vi "imp_test_v10.vi"() -> ()   [LabVIEW 2014]
uses:
  <vilib>/LabVIEW Targets/FPGA/cRIO/shared/nicrio_ModuleControls/nicrio_cRIO-9237_DataRatesRing.ctl
  <vilib>/LabVIEW Targets/FPGA/cRIO/shared/nicrio_ModuleControls/nicrio_cRIO-9237_ExcitationVoltageRing.ctl
  <vilib>/rvi/FXPMathLib/FxpSinAndCos/subVIs/nifxpmath_SinAndCos_SimConfig.ctl
  <vilib>/rvi/Emulation/niFpgaGetClockAttributes.vi
  <vilib>/rvi/Emulation/niFpgaSctlEmulationGetInTimedLoop.vi
  <vilib>/rvi/Emulation/niFpgaEmulationReportErrorSimple.vi
  <vilib>/rvi/Emulation/niFpgaProcessEmulError.vi
  <vilib>/rvi/interface/RandomDataEmulation/nirviRandomDataMultiElementFPGAFIFO.vi
  <instcachedir>/0/nirviRandomDataMultiElementFPGAFIFO_AD0CFC12EF974623A9C2E4184BC062B2.lvgen/nirviRandomDataMultiElementFPGAFIFO_AD0CFC12EF974623A9C2E4184BC062B2_010.vi
  <vilib>/rvi/interface/RandomDataEmulation/niFpgaRandomDataHandleErrors.vi
  <vilib>/rvi/Emulation/niFpgaCriticalErrorInLSC.vi
  <vilib>/rvi/FXPMathLib/FxpSinAndCos/simVIs/DllFxpSinAndCosTemp_sub.vi
  <vilib>/rvi/eio/common/nirviEmuTemplateMethod_errors.vi
  <vilib>/rvi/eio/common/nirviEmuTemplatePropertySet_errors.vi
  <vilib>/rvi/DataTransferAndStorage/Container/XNode/niFpgaContainer.xnode
  <vilib>/rvi/interface/RandomDataEmulation/nirviRandomDataFpgaMultiElementTemplate.vi
  <vilib>/rvi/FXPMathLib/FxpSinAndCos/XNode/nifxpmath_SinAndCos.xnode
  <vilib>/eio/EIONode/EIONode.xnode
  <vilib>/rvi/Analysis/measure/butterworth/XNode/niFpgaButterworthFilter.xnode
  <vilib>/eio/EIOPropertyNode/EIOPropertyNode.xnode
  <vilib>/rvi/eio/common/nirviEmuTemplatePropertyGet_errors.vi
  <vilib>/rvi/eio/common/nirviEmuTemplatePropertyGet_noerrors.vi
  <vilib>/rvi/eio/common/nirviEmuTemplatePropertySet_noerrors.vi
panel:
  in  "F_Threshold_p":fxp<+,12,4>
  in  "F_Threshold_y":fxp<+,12,4>
  out "omega_y (Mavg)":fxp<+/-,36,13>
  out "Dy_d (Mavg)":fxp<+/-,36,13>
  out "omega_p (Mavg)":fxp<+/-,36,13>
  out "Dp_d (Mavg)":fxp<+/-,36,13>
  out "omega_p2 (Mavg)":fxp<+/-,36,14>
  out "Dp2_d (Mavg)":fxp<+/-,36,14>
  out "omega_y2 (Mavg)":fxp<+/-,64,27>
  out "Dy2_d (Mavg)":fxp<+/-,36,14>
  in  "mt0_y2":u32
  in  "mt0_p2":u32
  out "Dy_d (Mavg w. f.)":fxp<+/-,36,14>
  out "Dp_d (Mavg w. f.)":fxp<+/-,36,14>
  in  "Dp_d (Mavg) coeff.":i32[](array[numeric])=[946630756, 63555534]
  in  "Dy_d (Mavg) coeff.":i32[](array[numeric])=[946630756, 63555534]
  out "omega_y (Mavg w. f.)":fxp<+/-,36,14>
  in  "omega_y(Mavg) coeff.":i32[](array[numeric])=[946630756, 63555534]
  out "omega_p (Mavg w. f)":fxp<+/-,36,14>
  in  "omega_P(Mavg) coeff.":i32[](array[numeric])=[946630756, 63555534]
  in  "FIFO":i16(ring) items=["Pitch_F+P", "imp ctrl", "Yaw_F+P"]
  out "PID (kHz)":fxp<+/-,20,10>
  in  "Set 6":bool
  in  "Set 5":bool
  in  "Set 4":bool
  in  "Set 3":bool
  in  "Set 2":bool
  in  "Set 1":bool
  out "Dy1_d (T)":fxp<+/-,36,13>
  out "omega_y1 (T)":fxp<+/-,36,13>
  out "Dp1_d (T)":fxp<+/-,36,13>
  out "omega_p1 (T)":fxp<+/-,36,13>
  out "Dy2_d (T)":fxp<+/-,36,13>
  out "Dp2_d (T)":fxp<+/-,36,13>
  out "omega_y2 (T)":fxp<+/-,36,13>
  out "omega_p2 (T)":fxp<+/-,36,13>
  out "mt_omega_y2":u32
  out "mt_omega_p2":u32
  out "rad_y2":fxp<+/-,33,20>
  out "D_y2":fxp<+/-,32,7>
  out "rad_y1":fxp<+/-,33,20>
  out "D_y1":fxp<+/-,32,7>
  out "Encoder Position_y1":i32
  out "Encoder Position_y2":i32
  out "Encoder Position_p2":i32
  out "D_p2":fxp<+/-,32,7>
  out "rad_p2":fxp<+/-,33,20>
  out "D_p1":fxp<+/-,32,7>
  out "rad_p1":fxp<+/-,33,20>
  out "Encoder Position_p1":i32
  in  "Mag. factor_y":fxp<+/-,20,3>
  in  "Mag. encoder_y":bool
  out "omega_y (rad/s)":fxp<+/-,36,13>
  out "Dy_d (mm/s)":fxp<+/-,36,13>
  in  "Vy. Est.":i16(ring) items=["T", "Mavg", "Mavg w. f."]
  out "omega_y1 (Mavg)":fxp<+/-,36,14>
  out "Dy1_d (Mavg)":fxp<+/-,36,14>
  in  "Dy_d_M_avg_Tc (uSec)":i32
  out "Dp1_d (Mavg)":fxp<+/-,36,14>
  out "omega_p1 (Mavg)":fxp<+/-,36,14>
  in  "Dp_d_M_avg_Tc (uSec)":i32
  out "Dp_d (T)":fxp<+/-,36,13>
  out "omega_p (T)":fxp<+/-,36,13>
  in  "Vp. Est.":i16(ring) items=["T", "Mavg", "Mavg w. f."]
  in  "Mag. factor_p":fxp<+/-,20,3>
  in  "Mag. encoder_p":bool
  in  "Belt_out_p":fxp<+/-,7,7>
  in  "Belt_in_p":fxp<+/-,6,6>
  in  "Belt_out_y":fxp<+/-,7,7>
  in  "Belt_in_y":fxp<+/-,6,6>
  out "Fp_dc":fxp<+/-,32,10>
  out "Fy_dc":fxp<+/-,32,10>
  in  "Zero_y":bool
  in  "Zero_p":bool
  in  "mt0_p1":u32
  in  "Encoder reset":bool
  out "fpt_d":fxp<+/-,36,18>
  out "Dp_error_dd":fxp<+/-,36,16>
  out "Dp_error_d":fxp<+/-,33,8>
  in  "Dp_dd coeff.":i32[](array[numeric])=[946630756, 63555534]
  out "Dp_dd":fxp<+/-,36,25>
  out "dFp_PID":fxp<+/-,36,18>
  in  "dFp_PID coeff.":i32[](array[numeric])=[946630756, 63555534]
  out "fpt_i":fxp<+/-,34,18>
  in  "Bv_p":fxp<+/-,22,8>
  in  "Kv_p":fxp<+/-,22,8>
  out "Dp_error":fxp<+/-,22,7>
  out "Dpr_sin":fxp<+/-,22,7>
  in  "Sin offset_p":fxp<+/-,22,7>
  in  "Sin magnitude_p":fxp<+/-,21,6>
  out "Dpr_sin_dd":fxp<+/-,35,20>
  out "Dpr_sin_d":fxp<+/-,33,15>
  out "Sin omega_p":fxp<+/-,34,9>
  in  "Sin wave freq._p (Hz)":fxp<+/-,32,6>
  in  "Dpr_step":fxp<+/-,22,7>
  out "Dpr_for":fxp<+/-,22,7>
  in  "Command_p":i16(ring) items=["Step", "Sine"]
  in  "Ki_p":fxp<+/-,30,9>
  out "Fp_PID":fxp<+/-,36,16>
  in  "fp_tolorance":fxp<+,22,6>
  out "fp_tilde":fxp<+/-,33,10>
  in  "Kd_p":fxp<+/-,30,9>
  in  "Kp_p":fxp<+/-,32,13>
  out "Fr_p":fxp<+/-,32,10>
  in  "S/F coeff_p":fxp<+/-,25,-10>
  in  "S/F coeff_y":fxp<+/-,25,-10>
  out "va_p":fxp<+/-,36,7>
  out "vb_p":fxp<+/-,37,8>
  out "vq_p_F":fxp<+/-,20,5> format="%.57g"
  out "vd_p_F":fxp<+/-,20,5>
  in  "dFp_add":bool
  in  "Stop motor_p":bool
  out "Force_p":fxp<+/-,32,10>
  in  "Strain selection_p":i16(ring) items=["Raw", "Avg.8", "Avg.8 w. filter"]
  out "Strain_p (Avg8 w. f)":fxp<+/-,36,8>
  in  "Strain_p Avg.8 coeff.":i32[](array[numeric])=[946630756, 63555534]
  out "Strain_p (Avg8)":fxp<+/-,36,4>
  out "Raw Strain_p":fxp<+/-,36,4>
  out "Mod6/AI3":fxp<+/-,36,4>
  in  "Strain gage reset_p":bool
  out "Dp_d (mm/s)":fxp<+/-,36,13>
  out "omega_p (rad/s)":fxp<+/-,36,13>
  out "mt_omega_p1":u32
  out "rad_p(NrTheta)":fxp<+/-,33,20>
  out "D_p(mm)":fxp<+/-,32,7>
  out "Encoder Position_p":i32
  in  "Encoder reset_p":bool
  out "Strain_y (Avg8 w. f)":fxp<+/-,36,8>
  in  "Strain_y Avg8 coeff.":i32[](array[numeric])=[-898916953, 1957103773, 3888751]
  out "Dyr_for":fxp<+/-,22,7>
  in  "Command_y":i16(ring) items=["Step", "Sine"]
  out "Strain_y (Avg8)":fxp<+/-,36,4>
  in  "Strain selection_y":i16(ring) items=["Raw", "Avg.8", "Avg.8 w. filter"]
  out "vb_y":fxp<+/-,38,8>
  out "va_y":fxp<+/-,38,8>
  out "fyt_d":fxp<+/-,36,18>
  out "Fr_y":fxp<+/-,32,10>
  in  "Bv_y":fxp<+/-,22,8>
  out "Dy_error_dd":fxp<+/-,36,16>
  out "Dy_error_d":fxp<+/-,33,8>
  in  "Kv_y":fxp<+/-,22,8>
  out "Dy_error":fxp<+/-,22,7>
  out "Dyr_sin_dd":fxp<+/-,35,20>
  out "Dyr_sin_d":fxp<+/-,33,15>
  out "Sin omega_y":fxp<+/-,34,9>
  out "Dyr_sin":fxp<+/-,22,7>
  in  "Sin offset_y":fxp<+/-,22,7>
  in  "Sin magnitude_y":fxp<+/-,21,6>
  out "Time now(s)":fxp<+,52,14>
  in  "Sin wave freq._y (Hz)":fxp<+/-,32,6>
  in  "Dyr_step":fxp<+/-,22,7>
  in  "Drive mode":i16(ring) items=["Backward", "Forward"]
  out "Dy_dd":fxp<+/-,36,25>
  in  "Dy_dd coeff.":i32[](array[numeric])=[946630756, 63555534]
  out "dFy_PID":fxp<+/-,36,18>
  in  "dFy_PID coeff.":i32[](array[numeric])=[946630756, 63555534]
  out "fyt_i":fxp<+/-,36,16>
  out "Fy_PID":fxp<+/-,36,16>
  in  "fy_tolorance":fxp<+,22,6>
  in  "Ki_y":fxp<+/-,30,9>
  in  "Kd_y":fxp<+/-,30,9>
  out "fy_tilde":fxp<+/-,32,10>
  in  "Kp_y":fxp<+/-,32,13>
  out "vq_y_F":fxp<+/-,20,5> format="%.57g"
  out "vd_y_F":fxp<+/-,20,5>
  in  "dFy_add":bool
  in  "Stop motor_y":bool
  out "Dy_d (T)":fxp<+/-,36,13>
  out "omega_y (T)":fxp<+/-,36,13>
  in  "mt0_y1":u32
  out "mt_omega_y1":u32
  out "rad_y(NrTheta)":fxp<+/-,33,20>
  out "D_y(mm)":fxp<+/-,32,7>
  out "Encoder Position_y":i32
  in  "Encoder reset_y":bool
  in  "Ini coe.":bool
  out "Loop rate (kHz)":fxp<+/-,36,7>
  out "Force_y":fxp<+/-,32,10>
  out "Raw Strain_y":fxp<+/-,36,4>
  in  "Strain gage reset_y":bool
  in  "Stop (Strain)":bool
  out "Mod6/AI2":fxp<+/-,36,4>
  in  "Excitation Voltage":T1 items=["2.5 Volts", "3.3 Volts", "5.0 Volts", "10.0 Volts", "External Excitation"]
  in  "Data Rate":T2=1 items=["50.000 kS/s (NI 9237)"=1, "25.000 kS/s (NI 9237)"=2, "16.667 kS/s (NI 9237)"=3, "12.500 kS/s (NI 9237)"=4, "10.000 kS/s (NI 9237)"=5, "8.333 kS/s (NI 9237)"=6, "7.143 kS/s (NI 9237)"=7, "6.250 kS/s (NI 9237)"=8, "5.556 kS/s (NI 9237)"=9, "5.000 kS/s (NI 9237)"=10, "4.545 kS/s (NI 9237)"=11, "4.167 kS/s (NI 9237)"=12, "3.846 kS/s (NI 9237)"=13, "3.571 kS/s (NI 9237)"=14, "3.333 kS/s (NI 9237)"=15, "3.125 kS/s (NI 9237)"=16, "2.941 kS/s (NI 9237)"=17, "2.778 kS/s (NI 9237)"=18, "2.632 kS/s (NI 9237)"=19, "2.500 kS/s (NI 9237)"=20, "2.381 kS/s (NI 9237)"=21, "2.273 kS/s (NI 9237)"=22, "2.174 kS/s (NI 9237)"=23, "2.083 kS/s (NI 9237)"=24, "2.000 kS/s (NI 9237)"=25, "1.923 kS/s (NI 9237)"=26, "1.852 kS/s (NI 9237)"=27, "1.786 kS/s (NI 9237)"=28, "1.724 kS/s (NI 9237)"=29, "1.667 kS/s (NI 9237)"=30, "1.613 kS/s (NI 9237)"=31]
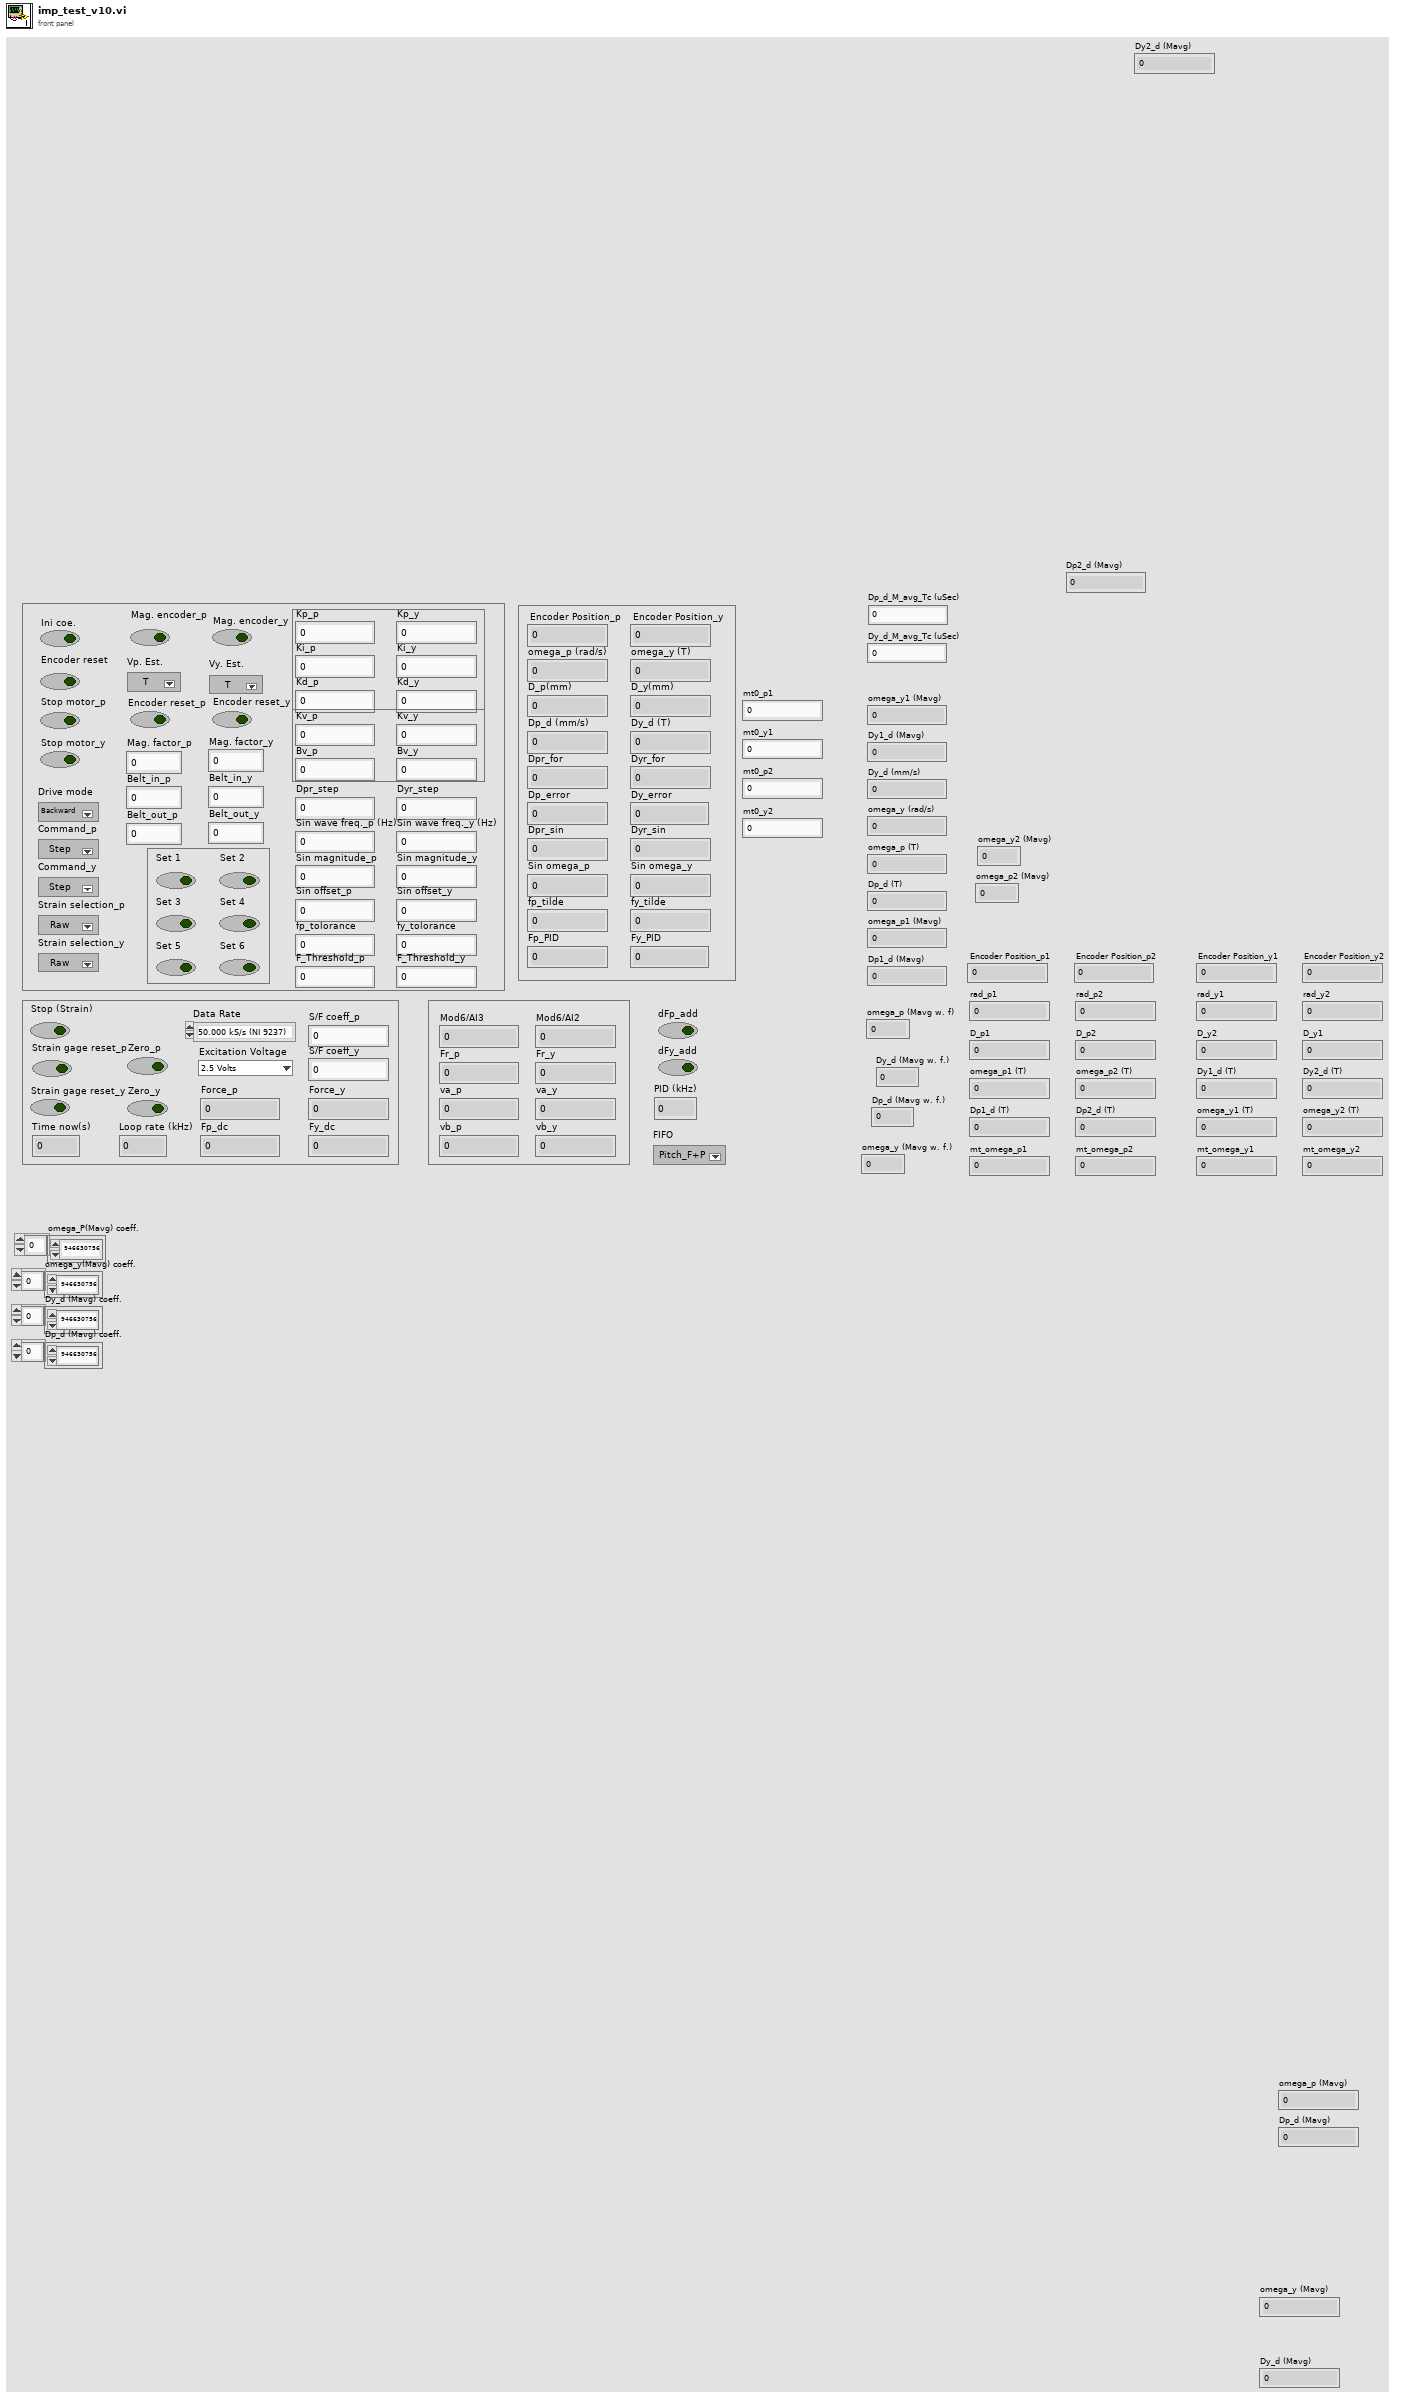
[diagram p1: front panel]
types:
  T1 = typedef "nicrio_cRIO-9237_ExcitationVoltageRing.ctl" = u8
  T2 = typedef "nicrio_cRIO-9237_DataRatesRing.ctl" = u8
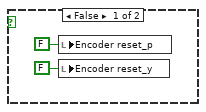
[diagram p12: hidden frame]
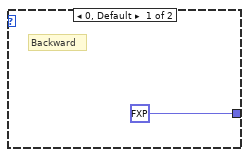
[diagram p13: hidden frame]
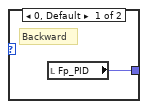
[diagram p14: hidden frame]
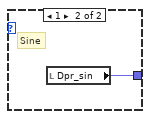
[diagram p15: hidden frame]
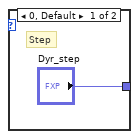
[diagram p16: hidden frame]
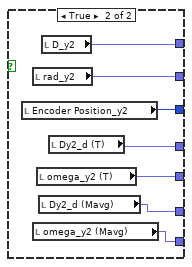
[diagram p17: hidden frame]
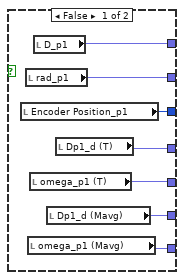
[diagram p18: hidden frame]
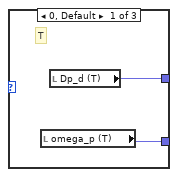
[diagram p19: hidden frame]
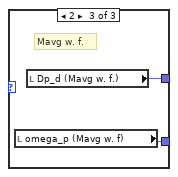
[diagram p20: hidden frame]
diagram:
  w2 = 25
  w5 = i16 25
  w13 = 25
  w16 = 25
  w21 = TRUE ("Half-Bridge Enable")
  # "rad_x2那邊:數據叫出來/8才會和馬達編碼器的rad一樣??"
  # "Encoder 4096ppr\nomega = 61359.2315154/mt\nomega0 = 2*pi/4096 (rad/s)"
  # "Encoder 800ppr\nomega = 314159.265359/mt\nomega0 = 2*pi/800 (rad/s)"
  # "v9\nKp改32/13\nKd改30/9\nKo改30/9"
  # "Resolutuin of Mag. Encoder = 4096*(F_mag)"
  # "use Mavg method to estimate omega or velocity from magnetic encoder"
  # "為什麼要寫兩個迴圈?\nv9後已修正"
  # "Dr_dd ?"
  # "Dr_d ?"
  n1 = xnode "FPGA I/O Property Node"("error in"=errorcluster {"status"=FALSE, "code"=0, "source"=""}, "Data Rate"="Data Rate", "Excitation Voltage"="Excitation Voltage") -> ("error out"=w26:errorcluster)  [unwired: 1 in, 1 out]
  n2 = xnode "FPGA I/O Property Node"("error in"=w26, "Half-Bridge Enable"=w21) -> ("error out"=w19:errorcluster)  [unwired: 1 in, 1 out]
  n3 = xnode "FPGA I/O Property Node"("Half-Bridge Enable"=w21) -> ("error out"=w18:errorcluster)  [unwired: 2 in, 1 out]
  n4 = Merge Errors(w19, w18) -> (w20:errorcluster)
  n5 = xnode "FPGA I/O Node"("error in"=w20, "Mod6/Start"=TRUE) -> ("error out"=w24:errorcluster)  [unwired: 1 in, 1 out]
  n6 = while "AO_p" {
    stop <- FALSE stop-if-true
    n7 = flat-sequence {
      frame #0 {
        n8 = local read "rad_p(NrTheta)"() -> (w41:fxp<+/-,33,20>)
        n9 = local read "vq_p_F"() -> (w42:fxp<+/-,20,5>)
        n10 = local read "vd_p_F"() -> (w44:fxp<+/-,20,5>)
        n11 = Select(t=fxp<+/-,20,5> 0.0, s="Stop motor_p", f=w44) -> (s? t:f=w33:fxp<+/-,20,5>)
        n12 = Select(t=fxp<+,1,1> 0.0, s="Stop motor_p", f=w42) -> (s? t:f=w32:fxp<+/-,20,5>)
        n13 = xnode "High Throughput Sine & Cosine"("x (pi)"=w41) -> ("sin(x)"=w35:fxp<+/-,16,2>, "cos(x)"=w34:fxp<+/-,16,2>)
        n14 = Negate(x=w32) -> (-x=w40:fxp<+/-,21,6>)
        n15 = Multiply(x=w33, y=w35) -> (x*y=w39:fxp<+/-,36,7>)
        n16 = Multiply(x=w33, y=w34) -> (x*y=w37:fxp<+/-,36,7>)
        n17 = Multiply(x=w34, y=w32) -> (x*y=w38:fxp<+/-,36,7>)
        n18 = Multiply(x=w35, y=w40) -> (x*y=w36:fxp<+/-,35,6>)
        n19 = Add(x=w39, y=w38) -> (x+y=→"vb_p":fxp<+/-,37,8>)
        n20 = Add(x=w37, y=w36) -> (x+y=→"va_p":fxp<+/-,36,7>)
      }
      frame #1 {
        n21 = local read "Encoder reset_p"() -> (w77:bool)
        n22 = local read "vb_p"() -> (w78:fxp<+/-,37,8>)
        n23 = local read "va_p"() -> (w79:fxp<+/-,36,7>)
        n24 = Select(t=fxp<+,2,2> 3.0, s=w77, f=w79) -> (s? t:f=w85:fxp<+/-,36,7>)
        n25 = Select(t=fxp<+,1,1> 0.0, s=w77, f=w78) -> (s? t:f=w84:fxp<+/-,37,8>)
        n26 = Multiply(x=w85, y=fxp<+/-,1,0> -0.5) -> (x*y=w80:fxp<+/-,36,6>)
        n27 = Multiply(x=w84, y=fxp<+/-,1,0> -0.5) -> (x*y=w81:fxp<+/-,36,6>)
        n28 = xnode "FPGA I/O Node"("Mod8/AO0"=w80, "Mod8/AO1"=w81) -> ()  [unwired: 2 in, 2 out]
      }
    }
  }
  n29 = while "AO_y" {
    stop <- FALSE stop-if-true
    n30 = flat-sequence {
      frame #0 {
        n31 = local read "rad_y(NrTheta)"() -> (w105:fxp<+/-,33,20>)
        n32 = local read "vd_y_F"() -> (w103:fxp<+/-,20,5>)
        n33 = local read "vq_y_F"() -> (w102:fxp<+/-,20,5>)
        n34 = Select(t=fxp<+/-,20,5> 0.0, s="Stop motor_y", f=w103) -> (s? t:f=w97:fxp<+/-,20,5>)
        n35 = Select(t=fxp<+/-,20,5> 0.0, s="Stop motor_y", f=w102) -> (s? t:f=w96:fxp<+/-,20,5>)
        n36 = xnode "High Throughput Sine & Cosine"("x (pi)"=w105) -> ("sin(x)"=w99:fxp<+/-,17,2>, "cos(x)"=w98:fxp<+/-,17,2>)
        n37 = Negate(x=w96) -> (-x=w95:fxp<+/-,21,6>)
        n38 = Multiply(x=w97, y=w99) -> (x*y=w94:fxp<+/-,37,7>)
        n39 = Multiply(x=w97, y=w98) -> (x*y=w92:fxp<+/-,37,7>)
        n40 = Multiply(x=w98, y=w96) -> (x*y=w93:fxp<+/-,37,7>)
        n41 = Multiply(x=w99, y=w95) -> (x*y=w91:fxp<+/-,36,6>)
        n42 = Add(x=w94, y=w93) -> (x+y=→"vb_y":fxp<+/-,38,8>)
        n43 = Add(x=w92, y=w91) -> (x+y=→"va_y":fxp<+/-,37,7>)
      }
      frame #1 {
        n44 = local read "Encoder reset_y"() -> (w138:bool)
        n45 = local read "va_y"() -> (w137:fxp<+/-,38,8>)
        n46 = local read "vb_y"() -> (w136:fxp<+/-,38,8>)
        n47 = Select(t=fxp<+,2,2> 3.0, s=w138, f=w137) -> (s? t:f=w142:fxp<+/-,38,8>)
        n48 = Select(t=fxp<+,1,1> 0.0, s=w138, f=w136) -> (s? t:f=w141:fxp<+/-,38,8>)
        n49 = Multiply(x=w142, y=fxp<+/-,1,0> -0.5) -> (x*y=w145:fxp<+/-,39,8>)
        n50 = Multiply(x=w141, y=fxp<+/-,1,0> -0.5) -> (x*y=w146:fxp<+/-,37,6>)
        n51 = xnode "FPGA I/O Node"("Mod8/AO2"=w145, "Mod8/AO3"=w146) -> ()  [unwired: 2 in, 2 out]
      }
    }
  }
  n52 = while "Selection" {
    stop <- FALSE stop-if-true
    # "T = Mag. encoder\nF = Motor encoder"
    n53 = case shown="2" "Strain selection_y" {
      tunnel: [w229 w230 w231] -> w182
      frame 0, Default {
        n54 = local read "Raw Strain_y"() -> (w229:fxp<+/-,36,4>)
      }
      frame 1 {
        n55 = local read "Strain_y (Avg8)"() -> (w230:fxp<+/-,36,4>)
      }
      frame 2 {
        n56 = local read "Strain_y (Avg8 w. f)"() -> (w231:fxp<+/-,36,8>)
      }
    }
    n57 = case shown="1" "Vp. Est." {
      tunnel: [w213 w214 w217] -> w165
      tunnel: [w212 w215 w216] -> w166
      frame 0, Default {
        # "T"
        n58 = local read "omega_p (T)"() -> (w213:fxp<+/-,36,13>)
        n59 = local read "Dp_d (T)"() -> (w212:fxp<+/-,36,13>)
      }
      frame 1 {
        # "Mavg"
        n60 = local read "omega_p (Mavg)"() -> (w214:fxp<+/-,36,13>)
        n61 = local read "Dp_d (Mavg)"() -> (w215:fxp<+/-,36,13>)
      }
      frame 2 {
        # "Mavg w. f."
        n62 = local read "omega_p (Mavg w. f)"() -> (w217:fxp<+/-,36,14>)
        n63 = local read "Dp_d (Mavg w. f.)"() -> (w216:fxp<+/-,36,14>)
      }
    }
    "Dp_d (mm/s)" <- w166
    "omega_p (rad/s)" <- w165
    n64 = Divide(x=w182, y="S/F coeff_y") -> (x/y=w175:fxp<+/-,32,10>)
    n65 = case shown="True" "Zero_y" {
      tunnel: w175 -> [_ w225]
      frame False {
      }
      frame True {
        "Fy_dc" <- w225
      }
    }
    n66 = local read "Fy_dc"() -> (w176:fxp<+/-,32,10>)
    n67 = Subtract(x=w175, y=w176) -> (x-y=→"Force_y":fxp<+/-,33,11>)
    n68 = case shown="2" "Strain selection_p" {
      tunnel: [w226 w227 w228] -> w180
      frame 0, Default {
        n69 = local read "Raw Strain_p"() -> (w226:fxp<+/-,36,4>)
      }
      frame 1 {
        n70 = local read "Strain_p (Avg8)"() -> (w227:fxp<+/-,36,4>)
      }
      frame 2 {
        n71 = local read "Strain_p (Avg8 w. f)"() -> (w228:fxp<+/-,36,8>)
      }
    }
    n72 = case shown="1" "Vy. Est." {
      tunnel: [w219 w221 w223] -> w168
      tunnel: [w218 w220 w222] -> w169
      frame 0, Default {
        # "T"
        n73 = local read "omega_y (T)"() -> (w218:fxp<+/-,36,13>)
        n74 = local read "Dy_d (T)"() -> (w219:fxp<+/-,36,13>)
      }
      frame 1 {
        # "Mavg"
        n75 = local read "omega_y (Mavg)"() -> (w220:fxp<+/-,36,13>)
        n76 = local read "Dy_d (Mavg)"() -> (w221:fxp<+/-,36,13>)
      }
      frame 2 {
        # "Mavg w. f."
        n77 = local read "omega_y (Mavg w. f.)"() -> (w222:fxp<+/-,36,14>)
        n78 = local read "Dy_d (Mavg w. f.)"() -> (w223:fxp<+/-,36,14>)
      }
    }
    "Dy_d (mm/s)" <- w168
    "omega_y (rad/s)" <- w169
    n79 = Divide(x=w180, y="S/F coeff_p") -> (x/y=w172:fxp<+/-,32,10>)
    n80 = case shown="True" "Zero_p" {
      tunnel: w172 -> [_ w224]
      frame False {
      }
      frame True {
        "Fp_dc" <- w224
      }
    }
    n81 = local read "Fp_dc"() -> (w170:fxp<+/-,32,10>)
    n82 = Subtract(x=w172, y=w170) -> (x-y=→"Force_p":fxp<+/-,33,11>)
    n83 = case shown="False" "Mag. encoder_y" {
      tunnel: [w190 w196] -> w156
      tunnel: [w189 w197] -> w157
      tunnel: [w188 w195] -> w159
      tunnel: [w186 w194] -> w153
      tunnel: [w187 w193] -> w152
      tunnel: [w185 w192] -> w148
      tunnel: [w184 w191] -> w147
      frame False {
        n84 = local read "Encoder Position_y1"() -> (w188:i32)
        n85 = local read "omega_y1 (Mavg)"() -> (w184:fxp<+/-,36,14>)
        n86 = local read "Dy1_d (Mavg)"() -> (w185:fxp<+/-,36,14>)
        n87 = local read "rad_y1"() -> (w190:fxp<+/-,33,20>)
        n88 = local read "omega_y1 (T)"() -> (w186:fxp<+/-,36,13>)
        n89 = local read "D_y1"() -> (w189:fxp<+/-,32,7>)
        n90 = local read "Dy1_d (T)"() -> (w187:fxp<+/-,36,13>)
      }
      frame True {
        n91 = local read "Encoder Position_y2"() -> (w195:i32)
        n92 = local read "rad_y2"() -> (w196:fxp<+/-,33,20>)
        n93 = local read "omega_y2 (Mavg)"() -> (w191:fxp<+/-,64,27>)
        n94 = local read "omega_y2 (T)"() -> (w194:fxp<+/-,36,13>)
        n95 = local read "Dy2_d (Mavg)"() -> (w192:fxp<+/-,36,14>)
        n96 = local read "D_y2"() -> (w197:fxp<+/-,32,7>)
        n97 = local read "Dy2_d (T)"() -> (w193:fxp<+/-,36,13>)
      }
    }
    "D_y(mm)" <- w157
    "rad_y(NrTheta)" <- w156
    "Encoder Position_y" <- w159
    "Dy_d (T)" <- w152
    "omega_y (T)" <- w153
    "Dy_d (Mavg)" <- w148
    "omega_y (Mavg)" <- w147
    n98 = case shown="True" "Mag. encoder_p" {
      tunnel: [w204 w211] -> w161
      tunnel: [w203 w210] -> w162
      tunnel: [w202 w209] -> w163
      tunnel: [w200 w208] -> w155
      tunnel: [w201 w207] -> w154
      tunnel: [w199 w205] -> w151
      tunnel: [w198 w206] -> w150
      frame False {
        n99 = local read "Encoder Position_p1"() -> (w202:i32)
        n100 = local read "rad_p1"() -> (w203:fxp<+/-,33,20>)
        n101 = local read "omega_p1 (Mavg)"() -> (w198:fxp<+/-,36,14>)
        n102 = local read "omega_p1 (T)"() -> (w200:fxp<+/-,36,13>)
        n103 = local read "D_p1"() -> (w204:fxp<+/-,32,7>)
        n104 = local read "Dp1_d (Mavg)"() -> (w199:fxp<+/-,36,14>)
        n105 = local read "Dp1_d (T)"() -> (w201:fxp<+/-,36,13>)
      }
      frame True {
        n106 = local read "Encoder Position_p2"() -> (w209:i32)
        n107 = local read "omega_p2 (Mavg)"() -> (w206:fxp<+/-,36,14>)
        n108 = local read "rad_p2"() -> (w210:fxp<+/-,33,20>)
        n109 = local read "D_p2"() -> (w211:fxp<+/-,32,7>)
        n110 = local read "Dp2_d (Mavg)"() -> (w205:fxp<+/-,36,14>)
        n111 = local read "omega_p2 (T)"() -> (w208:fxp<+/-,36,13>)
        n112 = local read "Dp2_d (T)"() -> (w207:fxp<+/-,36,13>)
      }
    }
    "D_p(mm)" <- w161
    "rad_p(NrTheta)" <- w162
    "Encoder Position_p" <- w163
    "Dp_d (T)" <- w154
    "omega_p (T)" <- w155
    "Dp_d (Mavg)" <- w151
    "omega_p (Mavg)" <- w150
  }
  n113 = while "Quadrature drive_y" {
    stop <- FALSE stop-if-true
    n114 = local read "Drive mode"() -> (w233:i16)
    n115 = case shown="1" w233 {
      tunnel: [w243 w244] -> w232
      frame 0, Default {
        # "Backward"
        n116 = local read "Fy_PID"() -> (w243:fxp<+/-,36,16>)
      }
      frame 1 {
        # "Forward"
        n117 = local read "Fr_y"() -> (w244:fxp<+/-,32,10>)
      }
    }
    n118 = local read "dFy_PID"() -> (w236:fxp<+/-,36,18>)
    n119 = local read "omega_y (rad/s)"() -> (w242:fxp<+/-,36,13>)
    n120 = Select(t=w236, s="dFy_add", f=fxp<+,1,1> 0.0) -> (s? t:f=w239:fxp<+/-,36,18>)
    n121 = call "Oriental_step_motor_PKP225.vi"("F_Threshold"="F_Threshold_y", "dFmr"=w239, "omega"=w242, "Fmr"=w232) -> ("vq_F"=→"vq_y_F":fxp<+/-,36,9>, "vd_F"=→"vd_y_F":fxp<+/-,36,9>)  [unwired: 6 in]
  }
  n122 = while "Encoder_p" {
    shift-right: [w282] -> _
    shift-left: _ -> [w281]
    shift-right: [w283] -> _
    shift-left: _ -> [w280]
    shift-right: [w277] -> _
    shift-left: _ -> [w279]
    shift-right: [w268] -> _
    shift-left: _ -> [w267]
    shift-right: [w269] -> _
    shift-left: _ -> [w270]
    shift-right: [w264] -> _
    shift-left: _ -> [w265]
    stop <- FALSE stop-if-true
    w260 = fxp<+/-,20,-5> 0.00048828125  # L/4096
    w258 = fxp<+/-,16,1> 0.0244140625  # 2*50/4096)
    w276 = fxp<+/-,20,-5> 0.002499997615814209  # L/800
    w250 = fxp<+/-,16,1> 0.125  # 2*50/800
    n123 = xnode "FPGA I/O Node"() -> ("Mod7/DIO0"=w285:bool, "Mod7/DIO1"=w284:bool)  [unwired: 2 in, 2 out]
    n124 = xnode "FPGA I/O Node"() -> ("Mod7/DIO4"=w272:bool, "Mod7/DIO5"=w271:bool)  [unwired: 2 in, 2 out]
    n125 = local read "Encoder reset_p"() -> (w266:bool)
    n126 = call "encoder_sub.vi"("A_pre"=w281, "B_pre"=w280, "Encoder Position_pre"=w279, "A input"=w285, "Encoder Position Reset"="Encoder reset_p", "B input"=w284) -> ("A"=w282:bool, "B"=w283:bool, "Encoder Position (Counts)"=w277:i32)  [unwired: 19 in]
    "Encoder Position_p1" <- w277
    n127 = call "encoder_sub.vi"("A_pre"=w267, "B_pre"=w270, "Encoder Position_pre"=w265, "A input"=w272, "Encoder Position Reset"=w266, "B input"=w271) -> ("A"=w268:bool, "B"=w269:bool, "Encoder Position (Counts)"=w264:i32)  [unwired: 19 in]
    "Encoder Position_p2" <- w264
    n128 = local read "Belt_in_p"() -> (w275:fxp<+/-,6,6>)
    n129 = local read "Belt_in_p"() -> (w261:fxp<+/-,6,6>)
    n130 = local read "Belt_out_p"() -> (w273:fxp<+/-,7,7>)
    n131 = To Fixed-Point(number=w264) -> (fixed-point=w246:fxp<+/-,32,32>)  [unwired: 1 in]
    n132 = To Fixed-Point(number=w277) -> (fixed-point=w251:fxp<+/-,32,32>)  [unwired: 1 in]
    n133 = local read "Belt_out_p"() -> (w263:fxp<+/-,7,7>)
    n134 = local read "Mag. factor_p"() -> (w257:fxp<+/-,20,3>)
    n135 = Divide(x=w260, y="Mag. factor_p") -> (x/y=w259:fxp<+/-,41,13>)
    n136 = Multiply(x=w276, y=w275) -> (x*y=w274:fxp<+/-,26,1>)
    n137 = Multiply(x=w259, y=w261) -> (x*y=w262:fxp<+/-,46,18>)
    n138 = Divide(x=w274, y=w273) -> (x/y=w253:fxp<+/-,33,1>)
    n139 = Divide(x=w262, y=w263) -> (x/y=w248:fxp<+/-,53,18>)
    n140 = Divide(x=w258, y=w257) -> (x/y=w245:fxp<+/-,37,5>)
    n141 = Multiply(x=w251, y=w250) -> (x*y=→"rad_p1":fxp<+/-,33,20>)
    n142 = Multiply(x=w248, y=w246) -> (x*y=→"D_p2":fxp<+/-,37,7>)
    n143 = Multiply(x=w246, y=w245) -> (x*y=→"rad_p2":fxp<+/-,46,16>)
    n144 = Multiply(x=w253, y=w251) -> (x*y=→"D_p1":fxp<+/-,32,7>)
  }
  n145 = while "Integral and derivative" {
    shift-right: [w341] -> _
    shift-left: _ -> [w340]
    shift-right: [w333] -> _
    shift-left: _ -> [w332]
    shift-right: [w343] -> _
    shift-left: _ -> [w344]
    shift-right: [w323] -> _
    shift-left: _ -> [w322]
    shift-right: [w309] -> _
    shift-left: _ -> [w312]
    shift-right: [w302] -> _
    shift-left: _ -> [w301]
    shift-right: [w296] -> _
    shift-left: _ -> [w295]
    shift-right: [w291] -> _
    shift-left: _ -> [w292]
    stop <- FALSE stop-if-true
    # "Pitch"
    # "Yaw"
    n146 = local read "Dp_d (mm/s)"() -> (w291:fxp<+/-,36,13>)
    n147 = local read "Dy_d (mm/s)"() -> (w323:fxp<+/-,36,13>)
    n148 = local read "Fp_PID"() -> (w296:fxp<+/-,36,16>)
    n149 = local read "fp_tilde"() -> (w313:fxp<+/-,33,10>)
    n150 = local read "fp_tolorance"() -> (w316:fxp<+,22,6>)
    n151 = local read "fy_tolorance"() -> (w319:fxp<+,22,6>)
    n152 = local read "fy_tilde"() -> (w345:fxp<+/-,32,10>)
    n153 = local read "Fy_PID"() -> (w343:fxp<+/-,36,16>)
    n154 = Subtract(x=w296, y=w295) -> (x-y=w300:fxp<+/-,37,17>)
    n155 = Subtract(x=w291, y=w292) -> (x-y=w293:fxp<+/-,37,14>)
    n156 = Absolute Value(x=w313) -> (abs(x)=w317:fxp<+,33,10>)
    n157 = Absolute Value(x=w345) -> (abs(x)=w347:fxp<+,32,10>)
    n158 = Subtract(x=w343, y=w344) -> (x-y=w331:fxp<+/-,37,17>)
    n159 = Subtract(x=w323, y=w322) -> (x-y=w325:fxp<+/-,36,11>)
    n160 = Greater?(x=w347, y=w319) -> (0:w348:bool)
    n161 = Greater?(x=w317, y=w316) -> (0:w315:bool)
    n162 = Multiply(x=fxp<+,7,10> 1000.0, y=w300) -> (x*y=w298:fxp<+/-,32,18>)
    n163 = Multiply(x=fxp<+,7,10> 1000.0, y=w293) -> (x*y=w289:fxp<+/-,36,21>)
    n164 = local read "Stop motor_y"() -> (w334:bool)
    n165 = local read "Stop motor_p"() -> (w304:bool)
    n166 = Select(t=w345, s=w348, f=fxp<+/-,33,11> 0.0) -> (s? t:f=w341:fxp<+/-,33,11>)
    n167 = Select(t=w313, s=w315, f=fxp<+,1,1> 0.0) -> (s? t:f=w309:fxp<+/-,33,10>)
    n168 = Multiply(x=fxp<+,7,10> 1000.0, y=w325) -> (x*y=w324:fxp<+/-,36,21>)
    n169 = xnode "Butterworth Filter"("input data"=w298, "scaled coefficients"="dFp_PID coeff.") -> ("output data"=→"dFp_PID":fxp<+/-,36,22>)  [unwired: 1 in]
    n170 = xnode "Butterworth Filter"("input data"=w289, "scaled coefficients"="Dp_dd coeff.") -> ("output data"=→"Dp_dd":fxp<+/-,36,25>)  [unwired: 1 in]
    n171 = Multiply(x=fxp<+,7,10> 1000.0, y=w331) -> (x*y=w328:fxp<+/-,32,18>)
    n172 = Add(x=w340, y=w341) -> (x+y=w346:fxp<+/-,34,12>)
    n173 = Multiply(x=w312, y=w309) -> (x*y=w311:fxp<+/-,34,12>)
    n174 = xnode "Butterworth Filter"("input data"=w324, "scaled coefficients"="Dy_dd coeff.") -> ("output data"=→"Dy_dd":fxp<+/-,36,25>)  [unwired: 1 in]
    n175 = Multiply(x=fxp<+/-,30,12> 0.000499725341796875, y=w346) -> (x*y=w339:fxp<+/-,34,10>)
    n176 = Multiply(x=fxp<+/-,30,12> 0.000499725341796875, y=w311) -> (x*y=w308:fxp<+/-,34,10>)
    n177 = xnode "Butterworth Filter"("input data"=w328, "scaled coefficients"="dFy_PID coeff.") -> ("output data"=→"dFy_PID":fxp<+/-,36,22>)  [unwired: 1 in]
    n178 = Select(t=fxp<+,1,1> 0.0, s=w334, f=fxp<+,1,1> 1.0) -> (s? t:f=w337:fxp<+,1,1>)
    n179 = Select(t=fxp<+,1,1> 0.0, s=w304, f=fxp<+,1,1> 1.0) -> (s? t:f=w306:fxp<+,1,1>)
    n180 = Add(x=w339, y=w332) -> (x+y=w338:fxp<+/-,36,16>)
    n181 = Add(x=w308, y=w301) -> (x+y=w307:fxp<+/-,36,16>)
    n182 = Multiply(x=w338, y=w337) -> (x*y=w333:fxp<+/-,34,18>)
    "fyt_i" <- w333
    n183 = Multiply(x=w307, y=w306) -> (x*y=w302:fxp<+/-,34,18>)
    "fpt_i" <- w302
    n184 = call "Wait"("Count(uSec)"=u32 1000) -> ()  [unwired: 1 out]
  }
  n185 = while {
    stop <- FALSE stop-if-true
    n186 = case shown="True" "Set 3" {
      frame False {
      }
      frame True {
        n187 = local write "fp_tolorance"(fxp<+,22,6> 3.0 ("fp_tolorance")) -> ()
        n188 = local write "Kp_p"(fxp<+/-,36,9> 100.0 ("Kp_p")) -> ()
      }
    }
    n189 = case shown="True" "Set 2" {
      frame False {
      }
      frame True {
        n190 = local write "fp_tolorance"(fxp<+,22,6> 1.5 ("fp_tolorance")) -> ()
        n191 = local write "Kp_p"(fxp<+/-,36,9> 50.0 ("Kp_p")) -> ()
      }
    }
    n192 = case shown="True" "Set 1" {
      frame False {
      }
      frame True {
        n193 = local write "fp_tolorance"(fxp<+,22,6> 3.0 ("fp_tolorance")) -> ()
        n194 = local write "Kp_p"(fxp<+/-,36,9> 50.0 ("Kp_p")) -> ()
      }
    }
    n195 = case shown="True" "Set 5" {
      frame False {
      }
      frame True {
        n196 = local write "fp_tolorance"(fxp<+,22,6> 3.0 ("fp_tolorance")) -> ()
        n197 = local write "Kp_p"(fxp<+/-,36,9> 150.0 ("Kp_p")) -> ()
      }
    }
    n198 = case shown="True" "Set 6" {
      frame False {
      }
      frame True {
        n199 = local write "fp_tolorance"(fxp<+,22,6> 1.5 ("fp_tolorance")) -> ()
        n200 = local write "Kp_p"(fxp<+/-,36,9> 150.0 ("Kp_p")) -> ()
      }
    }
    n201 = case shown="True" "Set 4" {
      frame False {
      }
      frame True {
        n202 = local write "fp_tolorance"(fxp<+,22,6> 1.5 ("fp_tolorance")) -> ()
        n203 = local write "Kp_p"(fxp<+/-,36,9> 100.0 ("Kp_p")) -> ()
      }
    }
  }
  n204 = while "Omega_p(T method)" {
    shift-right: [w432] -> _
    shift-left: _ -> [w430]
    shift-right: [w413] -> _
    shift-left: _ -> [w431]
    shift-right: [w428] -> _
    shift-left: _ -> [w429]
    shift-right: [w406] -> _
    shift-left: _ -> [w405]
    shift-right: [w401] -> _
    shift-left: _ -> [w403]
    shift-right: [w409] -> _
    shift-left: _ -> [w408]
    stop <- FALSE stop-if-true
    w420 = fxp<+/-,32,0> 0.3183098859153688  # L/2/pi
    w425 = fxp<+/-,32,0> 0.3183098859153688  # L/2/pi
    n205 = local read "Encoder Position_p1"() -> (w432:i32)
    n206 = local read "Encoder Position_p2"() -> (w406:i32)
    n207 = call "Tick Count4"() -> ("Tick Count(Ticks)"=w407:u32)
    n208 = call "omega_sub_Encoder_800ppr.vi"("mt0"="mt0_p1", "omega_pre"=w431, "ticks_m_pre"=w429, "ticks"=w407, "count_pre"=w430, "count"=w432) -> ("ticks_m"=w428:u32, "mt"=→"mt_omega_p1":u32, "omega"=w413:fxp<+/-,36,13>)  [unwired: 3 in]
    "omega_p1 (T)" <- w413
    n209 = call "omega_sub_Encoder_4096ppr.vi"("mt0"="mt0_p2", "omega_pre"=w403, "ticks_m_pre"=w408, "ticks"=w407, "count_pre"=w405, "count"=w406) -> ("ticks_m"=w409:u32, "mt"=→"mt_omega_p2":u32, "omega"=w401:fxp<+/-,36,13>)  [unwired: 3 in]
    n210 = local read "Mag. factor_p"() -> (w421:fxp<+/-,20,3>)
    n211 = local read "Belt_in_p"() -> (w418:fxp<+/-,6,6>)
    n212 = local read "Belt_out_p"() -> (w417:fxp<+/-,7,7>)
    n213 = Multiply(x=w425, y="Belt_in_p") -> (x*y=w423:fxp<+/-,38,6>)
    n214 = Multiply(x=w420, y=w418) -> (x*y=w419:fxp<+/-,38,6>)
    n215 = Divide(x=w423, y="Belt_out_p") -> (x/y=w414:fxp<+/-,20,1>)
    n216 = Divide(x=w401, y=w421) -> (x/y=w402:fxp<+/-,57,31>)
    "omega_p2 (T)" <- w402
    n217 = Divide(x=w419, y=w417) -> (x/y=w412:fxp<+/-,45,6>)
    n218 = Multiply(x=w412, y=w402) -> (x*y=→"Dp2_d (T)":fxp<+/-,36,13>)
    n219 = Multiply(x=w414, y=w413) -> (x*y=→"Dp1_d (T)":fxp<+/-,36,13>)
  }
  n220 = while "PD position controller_y" {
    stop <- FALSE stop-if-true
    n221 = case shown="1" "Drive mode" {
      tunnel: [fxp<+/-,62,19> 0.0 w438] -> w434
      frame 0, Default {
        # "Backward"
      }
      frame 1 {
        # "Forward"
        n222 = local read "Dy_error_d"() -> (w440:fxp<+/-,33,8>)
        n223 = local read "D_y(mm)"() -> (w445:fxp<+/-,32,7>)
        n224 = local read "Dyr_for"() -> (w437:fxp<+/-,22,7>)
        n225 = Subtract(x=w437, y=w445) -> (x-y=w444:fxp<+/-,33,8>)
        "Dy_error" <- w444
        n226 = Multiply(x=w444, y="Kv_y") -> (x*y=w442:fxp<+/-,54,15>)
        n227 = Multiply(x=w440, y="Bv_y") -> (x*y=w439:fxp<+/-,55,16>)
        n228 = Add(x=w442, y=w439) -> (x+y=w438:fxp<+/-,55,16>)
      }
    }
    "Fr_y" <- w434
  }
  n229 = while "Command type" {
    stop <- FALSE stop-if-true
    n230 = case shown="1" "Command_y" {
      tunnel: ["Dyr_step" w454] -> w449
      frame 0, Default {
        # "Step"
      }
      frame 1 {
        # "Sine"
        n231 = local read "Dyr_sin"() -> (w454:fxp<+/-,22,7>)
      }
    }
    "Dyr_for" <- w449
    n232 = case shown="0, Default" "Command_p" {
      tunnel: ["Dpr_step" w452] -> w447
      frame 0, Default {
        # "Step"
      }
      frame 1 {
        # "Sine"
        n233 = local read "Dpr_sin"() -> (w452:fxp<+/-,22,7>)
      }
    }
    "Dpr_for" <- w447
  }
  n234 = while "Sine wave gene" {
    stop <- FALSE stop-if-true
    w460 = fxp<+,20,3> 6.2831878662109375  # 2*pi
    w492 = fxp<+,20,3> 6.2831878662109375  # 2*pi
    n235 = local read "Time now(s)"() -> (w498:fxp<+,52,14>)
    n236 = local read "Sin wave freq._y (Hz)"() -> (w491:fxp<+/-,32,6>)
    n237 = Multiply(x="Sin wave freq._y (Hz)", y=fxp<+/-,10,3> 2.0) -> (x*y=w499:fxp<+/-,41,9>)
    n238 = local read "Sin magnitude_y"() -> (w489:fxp<+/-,21,6>)
    n239 = local read "Sin magnitude_y"() -> (w482:fxp<+/-,21,6>)
    n240 = local read "Sin omega_y"() -> (w485:fxp<+/-,34,9>)
    n241 = Multiply(x=w499, y=w498) -> (x*y=w497:fxp<+/-,41,19>)
    n242 = Square(x=w485) -> (x^2=w484:fxp<+,34,18>)
    n243 = xnode "High Throughput Sine & Cosine"("x (pi)"=w497) -> ("sin(x)"=w479:fxp<+/-,16,2>, "cos(x)"=w487:fxp<+/-,16,2>)
    n244 = Multiply(x=w492, y=w491) -> (x*y=w490:fxp<+/-,34,9>)
    "Sin omega_y" <- w490
    n245 = Negate(x=w484) -> (-x=w483:fxp<+/-,35,19>)
    n246 = Multiply(x=w490, y=w489) -> (x*y=w488:fxp<+/-,33,15>)
    n247 = Multiply(x=w483, y=w482) -> (x*y=w481:fxp<+/-,34,20>)
    n248 = Multiply(x=w487, y=w488) -> (x*y=→"Dyr_sin_d":fxp<+/-,33,15>)
    n249 = Multiply(x="Sin magnitude_y", y=w479) -> (x*y=w495:fxp<+/-,37,8>)
    n250 = Multiply(x=w479, y=w481) -> (x*y=→"Dyr_sin_dd":fxp<+/-,35,20>)
    n251 = Add(x=w495, y="Sin offset_y") -> (x+y=→"Dyr_sin":fxp<+/-,37,8>)
    n252 = local read "Sin wave freq._p (Hz)"() -> (w456:fxp<+/-,32,6>)
    n253 = local read "Time now(s)"() -> (w474:fxp<+,52,14>)
    n254 = local read "Sin magnitude_p"() -> (w457:fxp<+/-,21,6>)
    n255 = local read "Sin magnitude_p"() -> (w459:fxp<+/-,21,6>)
    n256 = local read "Sin omega_p"() -> (w458:fxp<+/-,34,9>)
    n257 = Multiply(x="Sin wave freq._p (Hz)", y=fxp<+/-,10,3> 2.0) -> (x*y=w478:fxp<+/-,42,9>)
    n258 = Multiply(x=w478, y=w474) -> (x*y=w475:fxp<+/-,41,19>)
    n259 = Square(x=w458) -> (x^2=w470:fxp<+,34,18>)
    n260 = xnode "High Throughput Sine & Cosine"("x (pi)"=w475) -> ("sin(x)"=w461:fxp<+/-,16,2>, "cos(x)"=w466:fxp<+/-,16,2>)
    n261 = Multiply(x=w460, y=w456) -> (x*y=w473:fxp<+/-,34,9>)
    "Sin omega_p" <- w473
    n262 = Negate(x=w470) -> (-x=w469:fxp<+/-,35,19>)
    n263 = Multiply(x=w473, y=w457) -> (x*y=w472:fxp<+/-,33,15>)
    n264 = Multiply(x=w469, y=w459) -> (x*y=w468:fxp<+/-,35,19>)
    n265 = Multiply(x=w466, y=w472) -> (x*y=→"Dpr_sin_d":fxp<+/-,33,15>)
    n266 = Multiply(x=w461, y=w468) -> (x*y=→"Dpr_sin_dd":fxp<+/-,35,20>)
    n267 = Multiply(x="Sin magnitude_p", y=w461) -> (x*y=w464:fxp<+/-,37,8>)
    n268 = Add(x=w464, y="Sin offset_p") -> (x+y=→"Dpr_sin":fxp<+/-,37,8>)
  }
  n269 = while "Time reset" {
    shift-right: [w571] -> _
    shift-left: _ -> [w572]
    shift-right: [w566] -> _
    shift-left: _ -> [w567]
    stop <- FALSE stop-if-true
    n270 = local read "Stop motor_y"() -> (w573:bool)
    n271 = call "Tick Count3"() -> ("Tick Count(uSec)"=w571:u32)
    n272 = Subtract(x=w571, y=w572) -> (x-y=w570:u32)
    n273 = Add(x=w567, y=w570) -> (x+y=w569:u32)
    n274 = Select(t=u32 0, s=w573, f=w569) -> (s? t:f=w566:u32)
    n275 = To Fixed-Point(number=w566) -> (fixed-point=w565:fxp<+,32,32>)  [unwired: 1 in]
    n276 = Multiply(x=fxp<+,20,-18> 1.0000003385357559e-06, y=w565) -> (x*y=→"Time now(s)":fxp<+,52,14>)
  }
  n277 = while "Ini" {
    stop <- FALSE stop-if-true
    n278 = case shown="True" "Ini coe." {
      frame False {
      }
      frame True {
        w581 = T2 20 items=["50.000 kS/s (NI 9237)"=1, "25.000 kS/s (NI 9237)"=2, "16.667 kS/s (NI 9237)"=3, "12.500 kS/s (NI 9237)"=4, "10.000 kS/s (NI 9237)"=5, "8.333 kS/s (NI 9237)"=6, "7.143 kS/s (NI 9237)"=7, "6.250 kS/s (NI 9237)"=8, "5.556 kS/s (NI 9237)"=9, "5.000 kS/s (NI 9237)"=10, "4.545 kS/s (NI 9237)"=11, "4.167 kS/s (NI 9237)"=12, "3.846 kS/s (NI 9237)"=13, "3.571 kS/s (NI 9237)"=14, "3.333 kS/s (NI 9237)"=15, "3.125 kS/s (NI 9237)"=16, "2.941 kS/s (NI 9237)"=17, "2.778 kS/s (NI 9237)"=18, "2.632 kS/s (NI 9237)"=19, "2.500 kS/s (NI 9237)"=20, "2.381 kS/s (NI 9237)"=21, "2.273 kS/s (NI 9237)"=22, "2.174 kS/s (NI 9237)"=23, "2.083 kS/s (NI 9237)"=24, "2.000 kS/s (NI 9237)"=25, "1.923 kS/s (NI 9237)"=26, "1.852 kS/s (NI 9237)"=27, "1.786 kS/s (NI 9237)"=28, "1.724 kS/s (NI 9237)"=29, "1.667 kS/s (NI 9237)"=30, "1.613 kS/s (NI 9237)"=31] ("Data Rate")
        w598 = i16 0 items=["Step", "Sine"] ("Command_p")
        w599 = i16 2 items=["Raw", "Avg.", "Avg. w. filter"] ("Strain selection_p")
        w600 = i16 0 items=["Step", "Sine"] ("Command_y")
        w601 = i16 2 items=["Raw", "Avg.", "Avg. w. filter"] ("Strain selection_y")
        w603 = fxp<+/-,25,-10> 5.851034075021744e-07  # S/F coeff_p
        w602 = fxp<+/-,25,-10> 1.0477961041033268e-06  # S/F coeff_y
        w609 = i16 0 items=["Backward", "Forward"] ("Drive mode")
        n279 = local write "Sin wave freq._y (Hz)"(fxp<+/-,32,6> 1.0 ("Sin wave freq. (Hz)")) -> ()
        n280 = local write "Sin magnitude_y"(fxp<+/-,22,7> 5.0 ("Sin magnitude")) -> ()
        n281 = local write "fy_tolorance"(fxp<+,22,6> 5.0 ("f_tolorance")) -> ()
        n282 = local write "Sin offset_y"(fxp<+/-,38,9> 0.0 ("Sin offset")) -> ()
        n283 = local write "Dyr_step"(fxp<+/-,22,7> 0.0 ("Dr")) -> ()
        n284 = local write "Kp_y"(fxp<+/-,36,9> 30.0 ("Kp")) -> ()
        n285 = local write "Kd_y"(fxp<+/-,36,9> 0.0 ("Kd")) -> ()
        n286 = local write "Kv_y"(fxp<+/-,22,8> 0.0 ("Kv")) -> ()
        n287 = local write "Bv_y"(fxp<+/-,22,8> 0.0 ("Bv")) -> ()
        n288 = local write "Ki_y"(fxp<+/-,36,9> 0.0 ("Ki")) -> ()
        n289 = local write "S/F coeff_p"(w603) -> ()
        n290 = local write "S/F coeff_y"(w602) -> ()
        n291 = local write "Data Rate"(w581) -> ()
        n292 = local write "dFy_add"(FALSE ("dF_add")) -> ()
        n293 = local write "dFp_add"(FALSE ("dFp_add")) -> ()
        n294 = local write "Sin wave freq._p (Hz)"(fxp<+/-,32,6> 1.0 ("Sin wave freq._p (Hz)")) -> ()
        n295 = local write "Sin magnitude_p"(fxp<+/-,21,6> 5.0 ("Sin magnitude_p")) -> ()
        n296 = local write "fp_tolorance"(fxp<+,22,6> 5.0 ("fp_tolorance")) -> ()
        n297 = local write "Sin offset_p"(fxp<+/-,22,7> 0.0 ("Sin offset_p")) -> ()
        n298 = local write "Dpr_step"(fxp<+/-,22,7> 0.0 ("Dpr_step")) -> ()
        n299 = local write "Kp_p"(fxp<+/-,36,9> 30.0 ("Kp_p")) -> ()
        n300 = local write "Kd_p"(fxp<+/-,36,9> 0.0 ("Kd_p")) -> ()
        n301 = local write "Kv_p"(fxp<+/-,22,8> 0.0 ("Kv_p")) -> ()
        n302 = local write "Bv_p"(fxp<+/-,22,8> 0.0 ("Bv_p")) -> ()
        n303 = local write "Ki_p"(fxp<+/-,36,9> 0.0 ("Ki_p")) -> ()
        n304 = local write "Strain selection_p"(w599) -> ()
        n305 = local write "Strain selection_y"(w601) -> ()
        n306 = local write "Command_p"(w598) -> ()
        n307 = local write "Command_y"(w600) -> ()
        n308 = local write "Drive mode"(w609) -> ()
        n309 = local write "Dp_d_M_avg_Tc (uSec)"(u32 1000 ("D_d_M_avg_Tc (uSec)")) -> ()
        n310 = local write "Dy_d_M_avg_Tc (uSec)"(1000 ("Dy_d_M_avg_Tc (uSec)")) -> ()
        n311 = local write "Belt_out_p"(fxp<+/-,7,7> 36.0 ("Belt_op")) -> ()
        n312 = local write "Belt_out_y"(fxp<+/-,7,7> 22.0 ("Belt_oy")) -> ()
        n313 = local write "Belt_in_p"(fxp<+/-,6,6> 14.0 ("Belt_mp")) -> ()
        n314 = local write "Belt_in_y"(fxp<+/-,6,6> 16.0 ("Belt_my")) -> ()
        n315 = local write "mt0_p1"(u32 628319 ("mt0_p1")) -> ()
        n316 = local write "mt0_p2"(u32 628319 ("mt0_p2")) -> ()
        n317 = local write "mt0_y1"(u32 628319 ("mt0_y1")) -> ()
        n318 = local write "mt0_y2"(u32 628319 ("mt0_y2")) -> ()
      }
    }
  }
  n319 = while "FIFO" {
    stop <- FALSE stop-if-true
    n320 = flat-sequence {
      frame #0 {
        n321 = call "Loop Timer"("Count(uSec)"=u32 1000) -> ()  [unwired: 1 out]
      }
      frame #1 {
        n322 = case shown="0" "FIFO" {
          tunnel: [w652 w668 w684] -> w636
          tunnel: [w651 w667 w683] -> w635
          tunnel: [w650 w666 w682] -> w634
          tunnel: [w649 w665 w681] -> w633
          tunnel: [w646 w664 w678] -> w631
          tunnel: [w647 w663 w679] -> w630
          tunnel: [w648 w662 w680] -> w629
          tunnel: [w644 w661 w676] -> w628
          tunnel: [w643 w660 w675] -> w627
          tunnel: [w642 w659 w674] -> w626
          tunnel: [w641 w658 w673] -> w625
          tunnel: [w640 w657 w672] -> w624
          tunnel: [w639 w656 w671] -> w623
          tunnel: [w638 w655 w670] -> w622
          tunnel: [w637 fxp<+,1,1> 0.0 ("element") w669] -> w621
          tunnel: [w645 fxp<+,1,1> 0.0 w677] -> w619
          frame 0 {
            # "Pitch"
            n323 = local read "omega_p2 (Mavg)"() -> (w637:fxp<+/-,36,14>)
            n324 = local read "omega_p1 (Mavg)"() -> (w646:fxp<+/-,36,14>)
            n325 = local read "Encoder Position_p1"() -> (w652:i32)
            n326 = local read "Encoder Position_p2"() -> (w651:i32)
            n327 = local read "D_p1"() -> (w650:fxp<+/-,32,7>)
            n328 = local read "D_p2"() -> (w649:fxp<+/-,32,7>)
            n329 = local read "omega_p1 (T)"() -> (w648:fxp<+/-,36,13>)
            n330 = local read "omega_p2 (T)"() -> (w647:fxp<+/-,36,13>)
            n331 = local read "rad_p1"() -> (w645:fxp<+/-,33,20>)
            n332 = local read "rad_p2"() -> (w644:fxp<+/-,33,20>)
            n333 = local read "Force_p"() -> (w643:fxp<+/-,32,10>)
            n334 = local read "vb_p"() -> (w638:fxp<+/-,37,8>)
            n335 = local read "Fp_PID"() -> (w642:fxp<+/-,36,16>)
            n336 = local read "vd_p_F"() -> (w641:fxp<+/-,20,5>)
            n337 = local read "va_p"() -> (w639:fxp<+/-,36,7>)
            n338 = local read "vq_p_F"() -> (w640:fxp<+/-,20,5>)
          }
          frame 1, Default {
            # "imp ctrl"
            n339 = local read "D_y(mm)"() -> (w668:fxp<+/-,32,7>)
            n340 = local read "Raw Strain_y"() -> (w667:fxp<+/-,36,4>)
            n341 = local read "Strain_y (Avg8)"() -> (w666:fxp<+/-,36,4>)
            n342 = local read "Strain_y (Avg8 w. f)"() -> (w665:fxp<+/-,36,8>)
            n343 = local read "Force_y"() -> (w662:fxp<+/-,32,10>)
            n344 = local read "Dy_d (T)"() -> (w663:fxp<+/-,36,13>)
            n345 = local read "Fy_dc"() -> (w664:fxp<+/-,32,10>)
            n346 = local read "D_p(mm)"() -> (w661:fxp<+/-,32,7>)
            n347 = local read "Raw Strain_p"() -> (w660:fxp<+/-,36,4>)
            n348 = local read "Strain_p (Avg8)"() -> (w659:fxp<+/-,36,4>)
            n349 = local read "Strain_p (Avg8 w. f)"() -> (w658:fxp<+/-,36,8>)
            n350 = local read "Force_p"() -> (w657:fxp<+/-,32,10>)
            n351 = local read "Dp_d (mm/s)"() -> (w656:fxp<+/-,36,13>)
            n352 = local read "Fp_dc"() -> (w655:fxp<+/-,32,10>)
          }
          frame 2 {
            # "Yaw"
            n353 = local read "omega_y (Mavg w. f.)"() -> (w670:fxp<+/-,36,14>)
            n354 = local read "omega_y1 (Mavg)"() -> (w678:fxp<+/-,36,14>)
            n355 = local read "Dy1_d (Mavg)"() -> (w669:fxp<+/-,36,14>)
            n356 = local read "Encoder Position_y1"() -> (w684:i32)
            n357 = local read "Encoder Position_y2"() -> (w683:i32)
            n358 = local read "D_y1"() -> (w682:fxp<+/-,32,7>)
            n359 = local read "D_y2"() -> (w681:fxp<+/-,32,7>)
            n360 = local read "omega_y1 (T)"() -> (w680:fxp<+/-,36,13>)
            n361 = local read "omega_y2 (T)"() -> (w679:fxp<+/-,36,13>)
            n362 = local read "rad_y1"() -> (w677:fxp<+/-,33,20>)
            n363 = local read "rad_y2"() -> (w676:fxp<+/-,33,20>)
            n364 = local read "Force_y"() -> (w675:fxp<+/-,32,10>)
            n365 = local read "Raw Strain_y"() -> (w674:fxp<+/-,36,4>)
            n366 = local read "Strain_y (Avg8)"() -> (w673:fxp<+/-,36,4>)
            n367 = local read "Strain_y (Avg8 w. f)"() -> (w672:fxp<+/-,36,8>)
            n368 = local read "Dy_d (mm/s)"() -> (w671:fxp<+/-,36,13>)
          }
        }
        n369 = Build Array(w636, w635, w634, w633, w629, w630, w631, w619, w628, w627, w626, w625, w624, w623, w622, w621) -> (w620:fxp<+/-,64,32>[])
        n370 = xnode ("FIFO Write")("Element"=w620, "Timeout"=0) -> ()  [unwired: 1 in, 2 out]
      }
    }
  }
  n371 = while "PID force controller_y" {
    stop <- FALSE stop-if-true
    n372 = local read "Force_y"() -> (w686:fxp<+/-,32,10>)
    n373 = local read "fyt_d"() -> (w695:fxp<+/-,36,18>)
    n374 = local read "Fr_y"() -> (w687:fxp<+/-,32,10>)
    n375 = Subtract(x=w687, y=w686) -> (x-y=w685:fxp<+/-,33,11>)
    "fy_tilde" <- w685
    n376 = Absolute Value(x=w685) -> (abs(x)=w702:fxp<+,32,10>)
    n377 = local read "fyt_i"() -> (w691:fxp<+/-,36,16>)
    n378 = Multiply(x="Kp_y", y=w685) -> (x*y=w693:fxp<+/-,64,23>)
    n379 = Multiply(x="Kd_y", y=w695) -> (x*y=w694:fxp<+/-,64,27>)
    n380 = Multiply(x="Ki_y", y=w691) -> (x*y=w689:fxp<+/-,64,25>)
    n381 = Add(x=w693, y=w694) -> (x+y=w690:fxp<+/-,64,28>)
    n382 = Greater?(x=w702, y="fy_tolorance") -> (0:w700:bool)
    n383 = Add(x=w690, y=w689) -> (x+y=w688:fxp<+/-,64,29>)
    n384 = Select(t=w688, s=w700, f=fxp<+/-,51,14> 0.0) -> (s? t:f=→"Fy_PID":fxp<+/-,64,29>)
  }
  n385 = for {
    N: w2 -> [_]
    tunnel: [w705] -> w4 mode=indexing
    tunnel: [w704] -> w3 mode=indexing
    tunnel: [w704] -> w1
    n386 = local read "Dp_d_M_avg_Tc (uSec)"() -> (w704:i32)
    n387 = local read "Encoder Position_p2"() -> (w705:i32)
    n388 = call "Wait5"("Count(uSec)"=w704) -> ()  [unwired: 1 out]
  }
  n389 = while {
    tunnel: w24 -> [w750]
    tunnel: [w724] -> w17
    shift-right: [w748] -> _
    shift-left: _ -> [w749]
    shift-right: [w744] -> _
    shift-left: _ -> [w745]
    shift-right: [w739] -> _
    shift-left: _ -> [w738]
    shift-right: [w738] -> _
    shift-left: _ -> [w737]
    shift-right: [w737] -> _
    shift-left: _ -> [w736]
    shift-right: [w736] -> _
    shift-left: _ -> [w735]
    shift-right: [w735] -> _
    shift-left: _ -> [w734]
    shift-right: [w734] -> _
    shift-left: _ -> [w733]
    shift-right: [w733] -> _
    shift-left: _ -> [w732]
    tunnel: w24 -> [w728]
    shift-right: [w721] -> _
    shift-left: _ -> [w722]
    shift-right: [w717] -> _
    shift-left: _ -> [w716]
    shift-right: [w716] -> _
    shift-left: _ -> [w715]
    shift-right: [w715] -> _
    shift-left: _ -> [w714]
    shift-right: [w714] -> _
    shift-left: _ -> [w713]
    shift-right: [w713] -> _
    shift-left: _ -> [w712]
    shift-right: [w712] -> _
    shift-left: _ -> [w711]
    shift-right: [w711] -> _
    shift-left: _ -> [w710]
    stop <- w725 stop-if-true
    w719 = fxp<+,20,2> 2.115001678466797  # Gage Factor
    n390 = xnode "FPGA I/O Node"("error in"=w750) -> ("error out"=w724:errorcluster, "Mod6/AI2"=w746:fxp<+/-,24,-4>)  [unwired: 1 in, 1 out]
    n391 = xnode "FPGA I/O Node"("error in"=w728) -> ("error out"=w726:errorcluster, "Mod6/AI3"=w720:fxp<+/-,24,-4>)  [unwired: 1 in, 1 out]
    n392 = Or(x=w724, y="Stop (Strain)") -> (x .or. y?=w727:bool)
    n393 = Select(t=w720, s="Strain gage reset_p", f=w722) -> (s? t:f=w721:fxp<+/-,24,-4>)
    n394 = Select(t=w746, s="Strain gage reset_y", f=w749) -> (s? t:f=w748:fxp<+/-,24,-4>)
    n395 = Or(x=w727, y=w726) -> (x .or. y?=w725:bool)
    n396 = Subtract(x=w720, y=w721) -> (x-y=w718:fxp<+/-,30,-3>)
    "Mod6/AI3" <- w718
    n397 = Subtract(x=w746, y=w748) -> (x-y=w747:fxp<+/-,30,-3>)
    "Mod6/AI2" <- w747
    n398 = Multiply(x=w719, y=w747) -> (x*y=w739:fxp<+/-,41,6>)
    "Raw Strain_y" <- w739
    n399 = Multiply(x=w719, y=w718) -> (x*y=w717:fxp<+/-,50,-1>)
    "Raw Strain_p" <- w717
    n400 = call "average_v2.vi"("Numeric 8"=w710, "Numeric"=w717, "Numeric 7"=w711, "Numeric 2"=w716, "Numeric 6"=w712, "Numeric 5"=w713, "Numeric 4"=w714, "Numeric 3"=w715) -> ("Mean (8pt)"=w709:fxp<+/-,32,4>)  [unwired: 1 in, 2 out]
    "Strain_p (Avg8)" <- w709
    n401 = call "average_v2.vi"("Numeric 8"=w732, "Numeric"=w739, "Numeric 7"=w733, "Numeric 2"=w738, "Numeric 6"=w734, "Numeric 5"=w735, "Numeric 4"=w736, "Numeric 3"=w737) -> ("Mean (8pt)"=w731:fxp<+/-,32,4>)  [unwired: 1 in, 2 out]
    "Strain_y (Avg8)" <- w731
    n402 = call "Tick Count"() -> ("Tick Count(uSec)"=w744:u32)
    n403 = xnode "Butterworth Filter"("input data"=w709, "scaled coefficients"="Strain_p Avg.8 coeff.") -> ("output data"=→"Strain_p (Avg8 w. f)":fxp<+/-,36,8>)  [unwired: 1 in]
    n404 = xnode "Butterworth Filter"("input data"=w731, "scaled coefficients"="Strain_y Avg8 coeff.") -> ("output data"=→"Strain_y (Avg8 w. f)":fxp<+/-,32,4>)  [unwired: 1 in]
    n405 = Subtract(x=w744, y=w745) -> (x-y=w742:fxp<+/-,32,16>)
    n406 = Divide(x=fxp<+,7,10> 1000.0, y=w742) -> (x/y=→"Loop rate (kHz)":fxp<+/-,40,27>)
  }
  n407 = for {
    N: w5 -> [_]
    tunnel: [w769] -> w8 mode=indexing
    tunnel: [w768] -> w7 mode=indexing
    tunnel: [w767] -> w6
    n408 = local read "Dy_d_M_avg_Tc (uSec)"() -> (w767:i32)
    n409 = local read "Encoder Position_y2"() -> (w769:i32)
    n410 = call "Wait4"("Count(uSec)"=w767) -> ("Tick Count(uSec)"=w768:u32)
  }
  n411 = for {
    N: w13 -> [_]
    tunnel: [w772] -> w12 mode=indexing
    tunnel: [w771] -> w11 mode=indexing
    tunnel: ["Dy_d_M_avg_Tc (uSec)"] -> w10
    n412 = local read "Encoder Position_y1"() -> (w771:i32)
    n413 = call "Wait3"("Count(uSec)"="Dy_d_M_avg_Tc (uSec)") -> ("Tick Count(uSec)"=w772:u32)
  }
  n414 = for {
    N: w16 -> [_]
    tunnel: ["Dp_d_M_avg_Tc (uSec)"] -> w9
    tunnel: [w774] -> w15 mode=indexing
    tunnel: [w773] -> w14 mode=indexing
    n415 = local read "Encoder Position_p1"() -> (w773:i32)
    n416 = call "Wait2"("Count(uSec)"="Dp_d_M_avg_Tc (uSec)") -> ("Tick Count(uSec)"=w774:u32)
  }
  n417 = while "Omega_p2 (Mavg)" {
    shift-right: [w777] -> _
    shift-left: w4 -> [w798]
    shift-right: [w778] -> _
    shift-left: w3 -> [w796]
    shift-right: [w782] -> _
    shift-left: _ -> [w780]
    tunnel: w2 -> [w794]
    tunnel: w1 -> [w799]
    stop <- FALSE stop-if-true
    w783 = fxp<+/-,27,3> 3.1415926814079285  # pi
    w786 = fxp<+,32,0> 0.1953125  # 800/4096
    w791 = fxp<+/-,32,0> 0.3183098859153688  # L/2/pi
    n418 = call "Tick Count9"() -> ("Tick Count(uSec)"=w793:u32)
    n419 = Index Array(array=w796, index=0) -> (element=w795:i32)
    n420 = Index Array(array=w798, index=0) -> (element=w797:i32)
    n421 = Multiply(x=w794, y=w799) -> (x*y=w802:i32)
    n422 = Add(x=w802, y=w795) -> (x+y=w801:i32)
    n423 = Greater Or Equal?(x=w793, y=w801) -> (x >= y?=w800:bool)
    n424 = case shown="True" w800 {
      tunnel: w798 -> [w806 w821]
      tunnel: w797 -> [_ w813]
      tunnel: w796 -> [w807 w822]
      tunnel: w795 -> [_ w823]
      tunnel: w794 -> [_ w820]
      tunnel: w793 -> [_ w808]
      tunnel: [w806 w811] -> w777
      tunnel: [w807 w810] -> w778
      tunnel: [w805 w809] -> w782
      tunnel: w780 -> [w805 _]
      frame False {
      }
      frame True {
        n425 = local read "Encoder Position_p2"() -> (w812:i32)
        n426 = Subtract(x=w808, y=w823) -> (x-y=w824:u32)
        n427 = Insert Into Array(array=w822, new element=w808) -> (w826:i32[])  [unwired: 1 in]
        n428 = Subtract(x=w812, y=w813) -> (x-y=w817:i32)
        n429 = Insert Into Array(array=w821, index=w820, new element=w812) -> (w827:i32[])
        n430 = To Fixed-Point(number=w824) -> (fixed-point=w814:fxp<+,32,32>)  [unwired: 1 in]
        n431 = Multiply(x=w817, y=2500) -> (x*y=w818:i32)
        n432 = To Fixed-Point(number=w818) -> (fixed-point=w819:fxp<+/-,32,32>)  [unwired: 1 in]
        n433 = Delete From Array(array=w826, length=1, index=0) -> (array with subset deleted=w810:i32[])  [unwired: 1 out]
        n434 = Delete From Array(array=w827, length=1, index=0) -> (array with subset deleted=w811:i32[])  [unwired: 1 out]
        n435 = Divide(x=w819, y=w814) -> (x/y=w809:fxp<+/-,64,32>)
      }
    }
    n436 = local read "Mag. factor_p"() -> (w785:fxp<+/-,20,3>)
    n437 = local read "Belt_in_p"() -> (w788:fxp<+/-,6,6>)
    n438 = local read "Belt_out_p"() -> (w787:fxp<+/-,7,7>)
    n439 = Divide(x=w786, y=w785) -> (x/y=w776:fxp<+/-,32,1>)
    n440 = Multiply(x=w783, y=w782) -> (x*y=w784:fxp<+/-,64,35>)
    n441 = Multiply(x=w791, y=w788) -> (x*y=w792:fxp<+/-,38,6>)
    n442 = Multiply(x=w776, y=w784) -> (x*y=w779:fxp<+/-,64,36>)
    "omega_p2 (Mavg)" <- w779
    n443 = Divide(x=w792, y=w787) -> (x/y=w790:fxp<+/-,45,6>)
    n444 = Multiply(x=w790, y=w779) -> (x*y=→"Dp2_d (Mavg)":fxp<+/-,64,41>)
  }
  n445 = while "Omega_y1 (Mavg)" {
    tunnel: w13 -> [w848]
    shift-right: [w846] -> _
    shift-left: w12 -> [w851]
    shift-right: [w845] -> _
    shift-left: w11 -> [w847]
    shift-right: [w840] -> _
    shift-left: _ -> [w844]
    tunnel: w10 -> [w839]
    stop <- FALSE stop-if-true
    w833 = fxp<+/-,32,0> 0.3183098859153688  # L/2/pi
    w842 = fxp<+/-,27,3> 0.007853984832763672  # 2*pi/800
    n446 = call "Tick Count6"() -> ("Tick Count(uSec)"=w852:u32)
    n447 = Index Array(array=w851, index=0) -> (element=w850:u32)
    n448 = Index Array(array=w847, index=0) -> (element=w849:i32)
    n449 = Multiply(x=w848, y=w839) -> (x*y=w854:i32)
    n450 = Add(x=w854, y=w850) -> (x+y=w853:u32)
    n451 = Greater Or Equal?(x=w852, y=w853) -> (x >= y?=w843:bool)
    n452 = case shown="True" w843 {
      tunnel: w852 -> [_ w875]
      tunnel: w848 -> [_ w872]
      tunnel: w851 -> [w859 w874]
      tunnel: w850 -> [_ w873]
      tunnel: w849 -> [_ w869]
      tunnel: w847 -> [w858 w871]
      tunnel: [w857 w867] -> w840
      tunnel: [w859 w866] -> w846
      tunnel: [w858 w865] -> w845
      tunnel: w844 -> [w857 _]
      frame False {
      }
      frame True {
        # "count/s"
        n453 = local read "Encoder Position_y1"() -> (w868:i32)
        n454 = Subtract(x=w875, y=w873) -> (x-y=w876:u32)
        n455 = Insert Into Array(array=w874, new element=w875) -> (w878:u32[])  [unwired: 1 in]
        n456 = Subtract(x=w868, y=w869) -> (x-y=w863:i32)
        n457 = Insert Into Array(array=w871, index=w872, new element=w868) -> (w879:i32[])
        n458 = To Fixed-Point(number=w876) -> (fixed-point=w862:fxp<+,32,32>)  [unwired: 1 in]
        n459 = To Fixed-Point(number=w863) -> (fixed-point=w870:fxp<+/-,32,32>)  [unwired: 1 in]
        n460 = Divide(x=w862, y=fxp<+,32,32> 1000000.0) -> (x/y=w861:fxp<+/-,64,32>)
        n461 = Delete From Array(array=w878, length=1, index=0) -> (array with subset deleted=w866:u32[])  [unwired: 1 out]
        n462 = Delete From Array(array=w879, length=1, index=0) -> (array with subset deleted=w865:i32[])  [unwired: 1 out]
        n463 = Divide(x=w870, y=w861) -> (x/y=w867:fxp<+/-,64,65>)
      }
    }
    n464 = local read "Belt_in_y"() -> (w835:fxp<+/-,6,6>)
    n465 = Multiply(x=w842, y=w840) -> (x*y=w838:fxp<+/-,64,68>)
    n466 = local read "Belt_out_y"() -> (w836:fxp<+/-,7,7>)
    n467 = Multiply(x=w833, y=w835) -> (x*y=w834:fxp<+/-,38,6>)
    n468 = Multiply(x=fxp<+/-,2,2> 1.0 ("f"), y=w838) -> (x*y=w837:fxp<+/-,64,70>)
    "omega_y1 (Mavg)" <- w837
    n469 = Divide(x=w834, y=w836) -> (x/y=w832:fxp<+/-,45,6>)
    n470 = Multiply(x=w832, y=w837) -> (x*y=→"Dy1_d (Mavg)":fxp<+/-,64,75>)
  }
  n471 = while "Omega_p1 (Mavg)" {
    tunnel: w16 -> [w900]
    shift-right: [w898] -> _
    shift-left: w15 -> [w903]
    shift-right: [w897] -> _
    shift-left: w14 -> [w899]
    shift-right: [w896] -> _
    shift-left: _ -> [w895]
    tunnel: w9 -> [w893]
    stop <- FALSE stop-if-true
    w887 = fxp<+/-,27,3> 3.1415926814079285  # pi
    w886 = fxp<+/-,32,0> 0.3183098859153688  # L/2/pi
    n472 = call "Tick Count5"() -> ("Tick Count(uSec)"=w904:u32)
    n473 = Index Array(array=w903, index=0) -> (element=w902:u32)
    n474 = Index Array(array=w899, index=0) -> (element=w901:i32)
    n475 = Multiply(x=w900, y=w893) -> (x*y=w906:i32)
    n476 = Add(x=w906, y=w902) -> (x+y=w905:u32)
    n477 = Greater Or Equal?(x=w904, y=w905) -> (x >= y?=w894:bool)
    n478 = case shown="True" w894 {
      tunnel: w904 -> [_ w927]
      tunnel: w900 -> [_ w924]
      tunnel: w903 -> [w911 w926]
      tunnel: w902 -> [_ w925]
      tunnel: w901 -> [_ w921]
      tunnel: w899 -> [w910 w923]
      tunnel: [w909 w919] -> w896
      tunnel: [w911 w918] -> w898
      tunnel: [w910 w917] -> w897
      tunnel: w895 -> [w909 _]
      frame False {
      }
      frame True {
        n479 = local read "Encoder Position_p1"() -> (w920:i32)
        n480 = Subtract(x=w927, y=w925) -> (x-y=w928:u32)
        n481 = Subtract(x=w920, y=w921) -> (x-y=w913:i32)
        n482 = Insert Into Array(array=w926, new element=w927) -> (w930:u32[])  [unwired: 1 in]
        n483 = Insert Into Array(array=w923, index=w924, new element=w920) -> (w931:i32[])
        n484 = To Fixed-Point(number=w928) -> (fixed-point=w915:fxp<+,32,32>)  [unwired: 1 in]
        n485 = Multiply(x=w913, y=2500) -> (x*y=w914:i32)
        n486 = To Fixed-Point(number=w914) -> (fixed-point=w922:fxp<+/-,32,32>)  [unwired: 1 in]
        n487 = Delete From Array(array=w930, length=1, index=0) -> (array with subset deleted=w918:u32[])  [unwired: 1 out]
        n488 = Delete From Array(array=w931, length=1, index=0) -> (array with subset deleted=w917:i32[])  [unwired: 1 out]
        n489 = Divide(x=w922, y=w915) -> (x/y=w919:fxp<+/-,64,32>)
      }
    }
    n490 = local read "Belt_in_p"() -> (w891:fxp<+/-,6,6>)
    n491 = local read "Belt_out_p"() -> (w890:fxp<+/-,7,7>)
    n492 = Multiply(x=w887, y=w896) -> (x*y=w892:fxp<+/-,64,35>)
    n493 = Multiply(x=w886, y=w891) -> (x*y=w889:fxp<+/-,38,6>)
    n494 = Multiply(x=fxp<+/-,2,2> 1.0 ("f"), y=w892) -> (x*y=w885:fxp<+/-,64,37>)
    "omega_p1 (Mavg)" <- w885
    n495 = Divide(x=w889, y=w890) -> (x/y=w884:fxp<+/-,45,6>)
    n496 = Multiply(x=w884, y=w885) -> (x*y=→"Dp1_d (Mavg)":fxp<+/-,64,42>)
  }
  n497 = while "Omega_y2 (Mavg)" {
    shift-right: [w936] -> _
    shift-left: w7 -> [w956]
    shift-right: [w935] -> _
    shift-left: w8 -> [w958]
    tunnel: w6 -> [w954]
    tunnel: w5 -> [w952]
    shift-right: [w939] -> _
    shift-left: _ -> [w950]
    stop <- FALSE stop-if-true
    w941 = fxp<+/-,27,3> 0.007853984832763672  # 2*pi/800
    w943 = fxp<+,32,0> 0.1953125  # 800/4096
    w948 = fxp<+/-,32,0> 0.3183098859153688  # L/2/pi
    n498 = call "Tick Count8"() -> ("Tick Count(uSec)"=w957:u32)
    n499 = Index Array(array=w956, index=0) -> (element=w955:u32)
    n500 = Index Array(array=w958, index=0) -> (element=w953:i32)
    n501 = Multiply(x=w952, y=w954) -> (x*y=w960:i32)
    n502 = Add(x=w960, y=w955) -> (x+y=w959:u32)
    n503 = Greater Or Equal?(x=w957, y=w959) -> (x >= y?=w951:bool)
    n504 = case shown="True" w951 {
      tunnel: w958 -> [w963 w976]
      tunnel: w957 -> [_ w979]
      tunnel: w956 -> [w964 w978]
      tunnel: w955 -> [_ w977]
      tunnel: w953 -> [_ w966]
      tunnel: w952 -> [_ w975]
      tunnel: [w964 w974] -> w936
      tunnel: [w963 w973] -> w935
      tunnel: [w965 w968] -> w939
      tunnel: w950 -> [w965 _]
      frame False {
      }
      frame True {
        n505 = local read "Encoder Position_y2"() -> (w967:i32)
        n506 = Subtract(x=w979, y=w977) -> (x-y=w982:u32)
        n507 = Insert Into Array(array=w978, new element=w979) -> (w984:u32[])  [unwired: 1 in]
        n508 = Insert Into Array(array=w976, index=w975, new element=w967) -> (w985:i32[])
        n509 = Subtract(x=w967, y=w966) -> (x-y=w971:i32)
        n510 = To Fixed-Point(number=w982) -> (fixed-point=w981:fxp<+,32,32>)  [unwired: 1 in]
        n511 = To Fixed-Point(number=w971) -> (fixed-point=w972:fxp<+/-,32,32>)  [unwired: 1 in]
        n512 = Divide(x=w981, y=fxp<+,32,32> 1000000.0) -> (x/y=w970:fxp<+/-,64,32>)
        n513 = Delete From Array(array=w984, length=1, index=0) -> (array with subset deleted=w974:u32[])  [unwired: 1 out]
        n514 = Delete From Array(array=w985, length=1, index=0) -> (array with subset deleted=w973:i32[])  [unwired: 1 out]
        n515 = Divide(x=w972, y=w970) -> (x/y=w968:fxp<+/-,64,65>)
      }
    }
    n516 = local read "Mag. factor_y"() -> (w942:fxp<+/-,20,3>)
    n517 = local read "Belt_in_y"() -> (w945:fxp<+/-,6,6>)
    n518 = local read "Belt_out_y"() -> (w944:fxp<+/-,7,7>)
    n519 = Multiply(x=w941, y=w939) -> (x*y=w940:fxp<+/-,64,68>)
    n520 = Divide(x=w943, y=w942) -> (x/y=w934:fxp<+/-,32,1>)
    n521 = Multiply(x=w948, y=w945) -> (x*y=w949:fxp<+/-,38,6>)
    n522 = Multiply(x=w934, y=w940) -> (x*y=w937:fxp<+/-,64,69>)
    "omega_y2 (Mavg)" <- w937
    n523 = Divide(x=w949, y=w944) -> (x/y=w947:fxp<+/-,45,6>)
    n524 = Multiply(x=w947, y=w937) -> (x*y=→"Dy2_d (Mavg)":fxp<+/-,64,74>)
  }
  n525 = while "Quadrature drive_p" {
    stop <- FALSE stop-if-true
    n526 = local read "Drive mode"() -> (w989:i16)
    n527 = case shown="1" w989 {
      tunnel: [w999 w1000] -> w988
      frame 0, Default {
        # "Backward"
        n528 = local read "Fp_PID"() -> (w999:fxp<+/-,36,16>)
      }
      frame 1 {
        # "Forward"
        n529 = local read "Fr_p"() -> (w1000:fxp<+/-,32,10>)
      }
    }
    n530 = local read "dFp_PID"() -> (w992:fxp<+/-,36,18>)
    n531 = local read "omega_p (rad/s)"() -> (w996:fxp<+/-,36,13>)
    n532 = Select(t=w992, s="dFp_add", f=fxp<+,1,1> 0.0) -> (s? t:f=w995:fxp<+/-,36,18>)
    n533 = call "Oriental_step_motor_PKP225.vi"("F_Threshold"="F_Threshold_p", "dFmr"=w995, "omega"=w996, "Fmr"=w988) -> ("vq_F"=→"vq_p_F":fxp<+/-,36,9>, "vd_F"=→"vd_p_F":fxp<+/-,36,9>)  [unwired: 6 in]
  }
  n534 = while "PID force controller_p" {
    shift-right: [w1005] -> _
    shift-left: _ -> [w1004]
    stop <- FALSE stop-if-true
    n535 = local read "Force_p"() -> (w1017:fxp<+/-,32,10>)
    n536 = local read "fpt_d"() -> (w1013:fxp<+/-,36,18>)
    n537 = local read "Fr_p"() -> (w1018:fxp<+/-,32,10>)
    n538 = Subtract(x=w1018, y=w1017) -> (x-y=w1015:fxp<+/-,33,11>)
    "fp_tilde" <- w1015
    n539 = local read "fpt_i"() -> (w1009:fxp<+/-,34,18>)
    n540 = Multiply(x="Kp_p", y=w1015) -> (x*y=w1011:fxp<+/-,64,23>)
    n541 = Multiply(x="Kd_p", y=w1013) -> (x*y=w1012:fxp<+/-,64,27>)
    n542 = Absolute Value(x=w1015) -> (abs(x)=w1024:fxp<+,32,10>)
    n543 = Add(x=w1011, y=w1012) -> (x+y=w1007:fxp<+/-,64,28>)
    n544 = Multiply(x="Ki_p", y=w1009) -> (x*y=w1008:fxp<+/-,64,27>)
    n545 = call "Tick Count7"() -> ("Tick Count(uSec)"=w1005:u32)
    n546 = Add(x=w1007, y=w1008) -> (x+y=w1006:fxp<+/-,64,29>)
    n547 = Greater?(x=w1024, y="fp_tolorance") -> (0:w1021:bool)
    n548 = Subtract(x=w1005, y=w1004) -> (x-y=w1003:u32)
    n549 = Divide(x=u32 1000, y=w1003) -> (x/y=→"PID (kHz)":fxp<+/-,20,7>)
    n550 = Select(t=w1006, s=w1021, f=fxp<+,1,1> 0.0) -> (s? t:f=→"Fp_PID":fxp<+/-,64,29>)
  }
  n551 = while "PD position controller_p" {
    stop <- FALSE stop-if-true
    n552 = local read "Drive mode"() -> (w1027:i16)
    n553 = case shown="1" w1027 {
      tunnel: [fxp<+/-,62,19> 0.0 w1030] -> w1026
      frame 0, Default {
        # "Backward"
      }
      frame 1 {
        # "Forward"
        n554 = local read "D_p(mm)"() -> (w1037:fxp<+/-,32,7>)
        n555 = local read "Dp_error_d"() -> (w1029:fxp<+/-,33,8>)
        n556 = local read "Dpr_for"() -> (w1036:fxp<+/-,22,7>)
        n557 = Subtract(x=w1036, y=w1037) -> (x-y=w1035:fxp<+/-,33,8>)
        "Dp_error" <- w1035
        n558 = Multiply(x=w1035, y="Kv_p") -> (x*y=w1032:fxp<+/-,54,15>)
        n559 = Multiply(x=w1029, y="Bv_p") -> (x*y=w1031:fxp<+/-,55,16>)
        n560 = Add(x=w1032, y=w1031) -> (x+y=w1030:fxp<+/-,55,16>)
      }
    }
    "Fr_p" <- w1026
  }
  n561 = while "All switch" {
    stop <- FALSE stop-if-true
    n562 = case shown="True" "Encoder reset" {
      frame False {
        n563 = local write "Encoder reset_p"(FALSE ("Encoder reset_p")) -> ()
        n564 = local write "Encoder reset_y"(FALSE ("Encoder reset_y")) -> ()
      }
      frame True {
        n565 = flat-sequence {
          frame #0 {
            n566 = local write "Encoder reset_p"(TRUE ("Encoder reset_p")) -> ()
          }
          frame #1 {
            n567 = local write "Encoder reset_y"(TRUE ("Encoder reset_y")) -> ()
            n568 = local write "Encoder reset_p"(FALSE ("Encoder reset_p")) -> ()
          }
          frame #2 {
            n569 = local write "Encoder reset_y"(FALSE ("Encoder reset_y")) -> ()
          }
        }
      }
    }
  }
  n570 = while "Derivative" {
    stop <- FALSE stop-if-true
    n571 = local read "Dpr_sin_dd"() -> (w1054:fxp<+/-,35,20>)
    n572 = local read "Stop motor_y"() -> (w1060:bool)
    n573 = local read "Dyr_sin_dd"() -> (w1062:fxp<+/-,35,20>)
    n574 = local read "Dpr_sin_d"() -> (w1056:fxp<+/-,33,15>)
    n575 = local read "Stop motor_p"() -> (w1052:bool)
    n576 = local read "Dyr_sin_d"() -> (w1065:fxp<+/-,33,15>)
    n577 = local read "Dp_error"() -> (w1057:fxp<+/-,22,7>)
    n578 = local read "Dy_error"() -> (w1066:fxp<+/-,22,7>)
    n579 = local read "Dp_dd"() -> (w1055:fxp<+/-,36,25>)
    n580 = local read "Dy_dd"() -> (w1063:fxp<+/-,36,25>)
    n581 = Subtract(x=w1065, y=w1066) -> (x-y=w1064:fxp<+/-,34,16>)
    n582 = Subtract(x=w1062, y=w1063) -> (x-y=w1061:fxp<+/-,41,26>)
    n583 = Subtract(x=w1056, y=w1057) -> (x-y=w1049:fxp<+/-,34,16>)
    n584 = Subtract(x=w1054, y=w1055) -> (x-y=w1053:fxp<+/-,41,26>)
    n585 = Select(t=fxp<+,1,1> 0.0, s=w1060, f=w1064) -> (s? t:f=→"Dy_error_d":fxp<+/-,34,16>)
    n586 = Select(t=fxp<+/-,64,49> 0.0, s=w1060, f=w1061) -> (s? t:f=→"Dy_error_dd":fxp<+/-,64,49>)
    n587 = Select(t=fxp<+,1,1> 0.0, s=w1052, f=w1049) -> (s? t:f=→"Dp_error_d":fxp<+/-,34,16>)
    n588 = Select(t=fxp<+/-,41,26> 0.0, s=w1052, f=w1053) -> (s? t:f=→"Dp_error_dd":fxp<+/-,41,26>)
  }
  n589 = while "ft_d" {
    stop <- FALSE stop-if-true
    n590 = local read "Dy_error_dd"() -> (w1084:fxp<+/-,36,16>)
    n591 = local read "Dp_error_dd"() -> (w1075:fxp<+/-,36,16>)
    n592 = local read "Dy_error_d"() -> (w1086:fxp<+/-,33,8>)
    n593 = local read "Dp_error_d"() -> (w1077:fxp<+/-,33,8>)
    n594 = local read "Kv_p"() -> (w1078:fxp<+/-,22,8>)
    n595 = local read "Bv_p"() -> (w1076:fxp<+/-,22,8>)
    n596 = local read "Kv_y"() -> (w1087:fxp<+/-,22,8>)
    n597 = local read "Bv_y"() -> (w1085:fxp<+/-,22,8>)
    n598 = local read "Force_y"() -> (w1080:fxp<+/-,32,10>)
    n599 = Multiply(x=w1086, y=w1087) -> (x*y=w1082:fxp<+/-,55,16>)
    n600 = Multiply(x=w1084, y=w1085) -> (x*y=w1083:fxp<+/-,58,24>)
    n601 = Multiply(x=w1077, y=w1078) -> (x*y=w1073:fxp<+/-,55,16>)
    n602 = Multiply(x=w1075, y=w1076) -> (x*y=w1074:fxp<+/-,58,24>)
    n603 = local read "Force_p"() -> (w1071:fxp<+/-,32,10>)
    n604 = Add(x=w1082, y=w1083) -> (x+y=w1081:fxp<+/-,63,24>)
    n605 = Add(x=w1073, y=w1074) -> (x+y=w1072:fxp<+/-,63,24>)
    n606 = Subtract(x=w1081, y=w1080) -> (x-y=→"fyt_d":fxp<+/-,63,24>)
    n607 = Subtract(x=w1072, y=w1071) -> (x-y=→"fpt_d":fxp<+/-,63,24>)
  }
  n608 = while "Encoder_y" {
    shift-right: [w1126] -> _
    shift-left: _ -> [w1118]
    shift-right: [w1125] -> _
    shift-left: _ -> [w1117]
    shift-right: [w1116] -> _
    shift-left: _ -> [w1114]
    shift-right: [w1122] -> _
    shift-left: _ -> [w1119]
    shift-right: [w1121] -> _
    shift-left: _ -> [w1120]
    shift-right: [w1115] -> _
    shift-left: _ -> [w1113]
    stop <- FALSE stop-if-true
    w1103 = fxp<+/-,16,1> 0.0244140625  # 2*50/4096
    w1108 = fxp<+/-,20,-5> 0.00048828125  # L/4096
    w1111 = fxp<+/-,20,-5> 0.002499997615814209  # L/800
    w1093 = fxp<+/-,16,1> 0.125  # 2*50/800
    n609 = xnode "FPGA I/O Node"() -> ("Mod7/DIO2"=w1127:bool, "Mod7/DIO3"=w1128:bool)  [unwired: 2 in, 2 out]
    n610 = xnode "FPGA I/O Node"() -> ("Mod7/DIO6"=w1124:bool, "Mod7/DIO7"=w1123:bool)  [unwired: 2 in, 2 out]
    n611 = local read "Encoder reset_y"() -> (w1098:bool)
    n612 = call "encoder_sub.vi"("A_pre"=w1118, "B_pre"=w1117, "Encoder Position_pre"=w1114, "A input"=w1127, "Encoder Position Reset"="Encoder reset_y", "B input"=w1128) -> ("A"=w1126:bool, "B"=w1125:bool, "Encoder Position (Counts)"=w1116:i32)  [unwired: 19 in]
    "Encoder Position_y1" <- w1116
    n613 = call "encoder_sub.vi"("A_pre"=w1119, "B_pre"=w1120, "Encoder Position_pre"=w1113, "A input"=w1124, "Encoder Position Reset"=w1098, "B input"=w1123) -> ("A"=w1122:bool, "B"=w1121:bool, "Encoder Position (Counts)"=w1115:i32)  [unwired: 19 in]
    "Encoder Position_y2" <- w1115
    n614 = local read "Belt_in_y"() -> (w1106:fxp<+/-,6,6>)
    n615 = local read "Belt_in_y"() -> (w1110:fxp<+/-,6,6>)
    n616 = local read "Belt_out_y"() -> (w1104:fxp<+/-,7,7>)
    n617 = Divide(x=w1108, y="Mag. factor_y") -> (x/y=w1107:fxp<+/-,41,13>)
    n618 = local read "Belt_out_y"() -> (w1109:fxp<+/-,7,7>)
    n619 = To Fixed-Point(number=w1115) -> (fixed-point=w1090:fxp<+/-,32,32>)  [unwired: 1 in]
    n620 = local read "Mag. factor_y"() -> (w1102:fxp<+/-,20,3>)
    n621 = To Fixed-Point(number=w1116) -> (fixed-point=w1094:fxp<+/-,32,32>)  [unwired: 1 in]
    n622 = Multiply(x=w1107, y=w1106) -> (x*y=w1105:fxp<+/-,46,18>)
    n623 = Multiply(x=w1111, y=w1110) -> (x*y=w1112:fxp<+/-,26,1>)
    n624 = Divide(x=w1105, y=w1104) -> (x/y=w1092:fxp<+/-,53,18>)
    n625 = Divide(x=w1112, y=w1109) -> (x/y=w1096:fxp<+/-,33,1>)
    n626 = Divide(x=w1103, y=w1102) -> (x/y=w1089:fxp<+/-,37,5>)
    n627 = Multiply(x=w1092, y=w1090) -> (x*y=→"D_y2":fxp<+/-,37,7>)
    n628 = Multiply(x=w1094, y=w1093) -> (x*y=→"rad_y1":fxp<+/-,33,20>)
    n629 = Multiply(x=w1096, y=w1094) -> (x*y=→"D_y1":fxp<+/-,32,7>)
    n630 = Multiply(x=w1090, y=w1089) -> (x*y=→"rad_y2":fxp<+/-,46,16>)
  }
  n631 = while "Omega_y(T method)" {
    shift-right: [w1154] -> _
    shift-left: _ -> [w1155]
    shift-right: [w1141] -> _
    shift-left: _ -> [w1157]
    shift-right: [w1159] -> _
    shift-left: _ -> [w1160]
    shift-right: [w1132] -> _
    shift-left: _ -> [w1133]
    shift-right: [w1130] -> _
    shift-left: _ -> [w1129]
    shift-right: [w1136] -> _
    shift-left: _ -> [w1135]
    stop <- FALSE stop-if-true
    w1148 = fxp<+/-,32,0> 0.3183098859153688  # L/2/pi
    w1153 = fxp<+/-,32,0> 0.3183098859153688  # L/2/pi
    n632 = local read "Encoder Position_y1"() -> (w1154:i32)
    n633 = call "Tick Count2"() -> ("Tick Count(Ticks)"=w1134:u32)
    n634 = local read "Encoder Position_y2"() -> (w1132:i32)
    n635 = call "omega_sub_Encoder_800ppr.vi"("mt0"="mt0_y1", "omega_pre"=w1157, "ticks_m_pre"=w1160, "ticks"=w1134, "count_pre"=w1155, "count"=w1154) -> ("ticks_m"=w1159:u32, "mt"=→"mt_omega_y1":u32, "omega"=w1141:fxp<+/-,36,13>)  [unwired: 3 in]
    "omega_y1 (T)" <- w1141
    n636 = call "omega_sub_Encoder_4096ppr.vi"("mt0"="mt0_y2", "omega_pre"=w1129, "ticks_m_pre"=w1135, "ticks"=w1134, "count_pre"=w1133, "count"=w1132) -> ("ticks_m"=w1136:u32, "mt"=→"mt_omega_y2":u32, "omega"=w1130:fxp<+/-,36,13>)  [unwired: 3 in]
    n637 = local read "Belt_in_y"() -> (w1147:fxp<+/-,6,6>)
    n638 = local read "Mag. factor_y"() -> (w1149:fxp<+/-,20,3>)
    n639 = local read "Belt_out_y"() -> (w1145:fxp<+/-,7,7>)
    n640 = Multiply(x=w1153, y="Belt_in_y") -> (x*y=w1151:fxp<+/-,38,6>)
    n641 = Multiply(x=w1148, y=w1147) -> (x*y=w1146:fxp<+/-,38,6>)
    n642 = Divide(x=w1146, y=w1145) -> (x/y=w1139:fxp<+/-,45,6>)
    n643 = Divide(x=w1151, y="Belt_out_y") -> (x/y=w1142:fxp<+/-,20,1>)
    n644 = Divide(x=w1130, y=w1149) -> (x/y=w1138:fxp<+/-,57,31>)
    "omega_y2 (T)" <- w1138
    n645 = Multiply(x=w1142, y=w1141) -> (x*y=→"Dy1_d (T)":fxp<+/-,36,13>)
    n646 = Multiply(x=w1139, y=w1138) -> (x*y=→"Dy2_d (T)":fxp<+/-,36,13>)
  }
  n647 = xnode "FPGA I/O Node"("error in"=w17, "Mod6/Stop"=TRUE) -> ()  [unwired: 1 in, 2 out]
  n648 = while {
    stop <- FALSE stop-if-true
    n649 = local read "omega_y1 (Mavg)"() -> (w1169:fxp<+/-,36,14>)
    n650 = local read "omega_p1 (Mavg)"() -> (w1173:fxp<+/-,36,14>)
    n651 = local read "Dp1_d (Mavg)"() -> (w1165:fxp<+/-,36,14>)
    n652 = local read "Dy1_d (Mavg)"() -> (w1166:fxp<+/-,36,14>)
    n653 = xnode "Butterworth Filter"("input data"=w1169, "scaled coefficients"="omega_y(Mavg) coeff.") -> ("output data"=→"omega_y (Mavg w. f.)":fxp<+/-,36,18>)  [unwired: 1 in]
    n654 = xnode "Butterworth Filter"("input data"=w1173, "scaled coefficients"="omega_P(Mavg) coeff.") -> ("output data"=→"omega_p (Mavg w. f)":fxp<+/-,36,18>)  [unwired: 1 in]
    n655 = xnode "Butterworth Filter"("input data"=w1166, "scaled coefficients"="Dy_d (Mavg) coeff.") -> ("output data"=→"Dy_d (Mavg w. f.)":fxp<+/-,36,18>)  [unwired: 1 in]
    n656 = xnode "Butterworth Filter"("input data"=w1165, "scaled coefficients"="Dp_d (Mavg) coeff.") -> ("output data"=→"Dp_d (Mavg w. f.)":fxp<+/-,36,18>)  [unwired: 1 in]
  }
